vi "Text control 2 v1.7.vi"() -> ()   [LabVIEW 2016]
panel:
  in  "byte count":u32=64
  in  "Serial Settings:Serial End Mode for Reads":u16(ring)=2 items=["None", "LastBit", "TermChar"]
  in  "Timeout (ms)":u32=10000
  in  "Enable Termination\nChar (T)":bool=TRUE
  in  "Termination char\n(0xA = '\\n' = LF)\n(0xD = '\\r' = CR)":u8=13 format="%.0x"
  in  "flow control":u16(ring) items=["None"=0, "XON/XOFF"=1, "RTS/CTS"=2, "DTR/DSR"=4]
  in  "stop bits":u16(ring)=10 items=["1.0"=10, "1.5"=15, "2.0"=20]
  in  "parity":u16(ring) items=["None", "Odd", "Even", "Mark", "Space"]
  in  "data bits":u16=8 min=5 max=8 step=1
  in  "VISA resource name":refnum<visa-resource-name>="COM6"
  in  "baud rate":u32=9600
  out "Serial output":string
  out "error out":errorcluster
  in  "Units":bool
  out "Elapsed Time":dbl caption="Elapsed Time (s)"
  out "Ion vs time":cluster{"Y data in":dbl[], "X data in":dbl[]}[](graph)
  out "Ig":dbl format="%.2e"
  out "Id":dbl format="%.2e"
  out "Is":dbl format="%.2e"
  out "I vs Vg":cluster{"Y data in":dbl[], "X data in":dbl[]}[](graph)
  in  "Panel Controls 2":T1={"Emergency Stop"=refnum, "TransGraph Max"=1e-05, "Text/Graph (text=false)"=TRUE, "TransGraph Min"=1e-11} {"TransGraph Min" format="%.2e"; "TransGraph Max" format="%.2e"}
  out "Currently running:":string="#output s 0 0 0 -0.008 0.008 0.002"
  in  "Lines left to run:":string
  in  "Standby":T2
  in  "Full Reset":bool
  in  "SMU4":cluster{"on/off":bool, "Voltage":dbl} {"Voltage" min=-100.0 max=100.0 format="%.2f"}
  in  "Source/Drain Range":u8(slide)=6 max=11 scale=0.0..11.0
  in  "Source/Drain\nRange mode":u16(ring) items=["Auto", "Limited", "Fixed"]
  in  "Gate Range":u8(slide)=6 max=11 scale=0.0..11.0
  in  "Gate Range\nmode":u16(ring) items=["Auto", "Limited", "Fixed"]
  in  "Gate":T3={"Gate Start"=0.0, "Gate Stop"=2.0, "Gate Step (linear only)"=1.0, "Gate Compliance"=0.0001, "Gate PComp"=0.0, "Range mode"=0, "Range"=6} {"Range" max=11 scale=0.0..11.0; "Range mode" items=["Auto", "Limited", "Fixed"]; "Gate PComp" format="%^.2e"; "Gate Compliance" format="%^.2e"; "Gate Step (linear only)" format="%^.4e"; "Gate Stop" format="%^.4e"; "Gate Start" format="%^.4e"}
  in  "Drain 2":T4={"Drain Start"=0.0, "Drain Stop"=2.0, "Drain Compliance"=0.0001, "Drain Step"=1.0, "Drain PComp"=0.0, "Range mode"=0, "Range"=6} {"Range" max=11 scale=0.0..11.0; "Range mode" items=["Auto", "Limited", "Fixed"]; "Drain PComp" format="%^.2e"; "Drain Step" format="%^.4e"; "Drain Compliance" format="%^.2e"; "Drain Stop" format="%^.4e"; "Drain Start" format="%^.4e"}
  in  "Timings 2":T5={"integration time"=0, "Short/Long integration time"=0.00064, "hold time (sec)"=0.0, "delay time (sec)"=0.0, "Step Time (0 disables)"=0.0, "sweep method"=0, "Pulse period"=0.005, "Base voltage"=0.0, "Pulse width"=0.0005} {"Pulse width" min=0.0005 max=0.1 step=0.0001 format="%.4f"; "Base voltage" format="%^.4e"; "Pulse period" min=0.005 max=1.0 step=0.0001 format="%.4f"; "sweep method" items=["Continuous", "Pulsed"]; "Step Time (0 disables)" format="%.2f"; "delay time (sec)" format="%.4f"; "hold time (sec)" format="%.4f"; "Short/Long integration time" format="%^.0e"; "integration time" scale=0.0..2.0}
  in  "Panel Controls":T6={"Emergency Stop"=refnum, "TransGraph Max"=1e-05, "Text/Graph (text=false)"=TRUE} {"TransGraph Max" format="%.2e"}
  in  "Interrupt run":bool
  in  "Drain: Compliance":dbl=0.001 format="%.8f"
  in  "Gate: Compliance":dbl=0.001 format="%.8f"
  out "Path":path=path "C:/users/rlp38/09Apr2009LTtesting/test2.txt"
  in  "hold time /s":dbl format="%.2f"
  in  "delay time /s":dbl format="%.2f"
  in  "integration time":u32(slide) max=2 step=1 scale=0.0..2.0
  in  "Integration time (short)":dbl=0.0019 min=8e-05 max=0.0019 step=8e-05 format="%^.0e"
  in  "Integration time (long)":dbl=0.32 min=0.04 max=2.0 step=0.02 format="%.2f"
  in  "Step delay /s":dbl format="%.2f"
  in  "Program":string="#pulsedstressV d 0.03 20 0 0.5 0.0827 5\n#\n#itime s\n#gaterangemode l\n#drainrangemode l\n#pulsed on 0.05 0 0.02\n#transfer d 1 -1 -0.1 -1 -1 0\n#wait-min 1\n#transfer d 1 -1 -0.1 -1 -1 0\n#output d 0 -1 -0.5 0 -1 -0.1\n#transfer d -10 40 1 5 40 35\n#transfer d -10 40 1 5 40 35\n#output d 0 40 20 0 40 1\n#\n#\n#sample 1 0.008 221 6 0.003\n#samplei 400e-6 200 6 0.002 0.1\n#vsu2pulse -10 4\n#\n#stressV 0.016 0.03 2e-4 0.1e-3 11\n#stressI 220e-7 0.08 15\n#transfer s -1 1 0.5 -0.005 0.005 0.005\n#output s 0 0 0 -0.008 0.008 0.002\n"
  # "Syntax:\nitime [s|m|l]\ngaterangemode [a|l|f]\ndrainrangemode [a|l|f]\npulsed [on|off] PulsePeriod(sec) PulseBaseVoltage PulseONWidth(sec)\nstandby [on l off]\nwait NumMilliseconds\nwait-min NumMinutes\n# texthere = comment\ntransfer [s|d] VgStart VgStop VgStep VdStart VdStop VdStep\noutput [s|d] VgStart VgStop VgStep VdStart VdStop VdStep\nsample Vg Vd NumSamples Time(s) SampleInterval(s)\nsamplei Idg NumSamples Time(s) SampleInterval(s) VDGcompliance\n# if in doubt use SampleInterval(s) = 0.004\nstressV VG VD IGcompliance IDcompliance Duration(sec)\nstressI IDG VDGcompliance Duration(sec)\nvsu2pulse Bias Duration(s)\npulsedstressV [s|d] VEstop VgON VgOFF Period(s) PulseONwidth(s) Vd\nsample-fpp Vg Vd NumSamples Time\nresample-fpp Vg Vd\ntransfer-fpp [s|d] VgStart VgStop VgStep VdStart VdStop VdStep\noutput-fpp [s|d] VgStart VgStop VgStep VdStart VdStop VdStep\nserial SerialPortCommand"
  # "Time"
  # "Sec"
  # "Min"
  # "100 samples is approx 13s with medium integration"
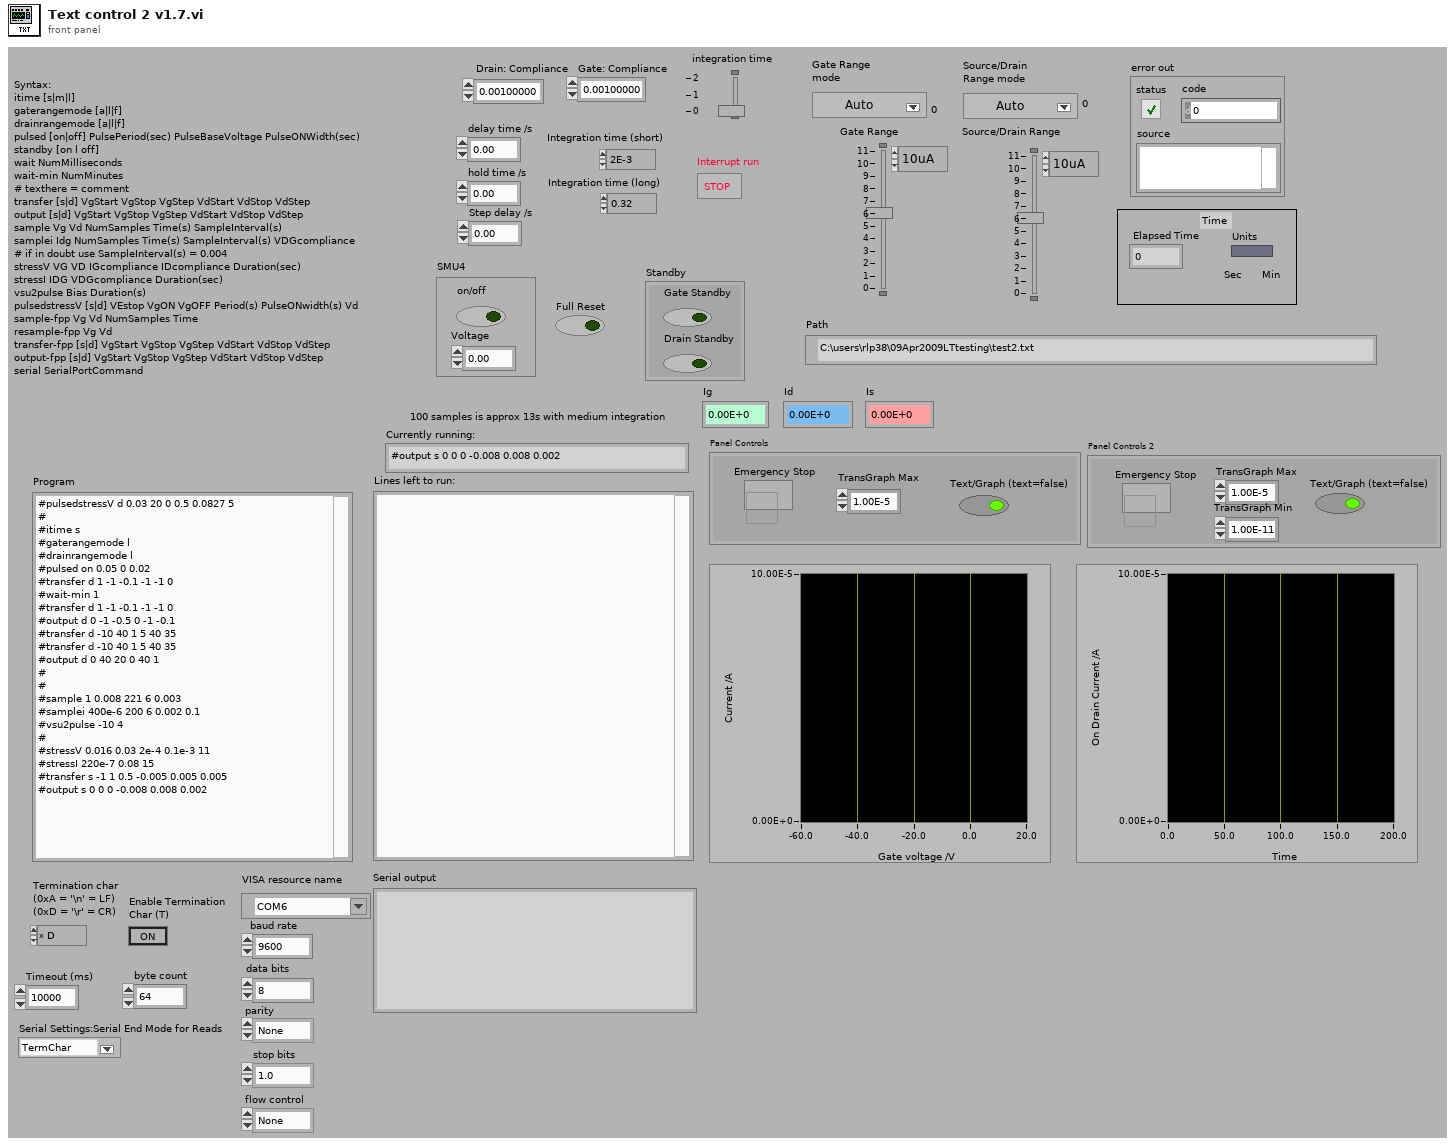
[diagram p1: front panel]
types:
  T1 = cluster{"Emergency Stop":refnum<vi>, "TransGraph Max":dbl, "Text/Graph (text=false)":bool, "TransGraph Min":dbl}
  T2 = cluster{"Gate Standby":bool, "Drain Standby":bool}
  T3 = cluster{"Gate Start":dbl, "Gate Stop":dbl, "Gate Step (linear only)":dbl, "Gate Compliance":dbl, "Gate PComp":dbl, "Range mode":u16, "Range":u8}
  T4 = cluster{"Drain Start":dbl, "Drain Stop":dbl, "Drain Compliance":dbl, "Drain Step":dbl, "Drain PComp":dbl, "Range mode":u16, "Range":u8}
  T5 = cluster{"integration time":u32, "Short/Long integration time":dbl, "hold time (sec)":dbl, "delay time (sec)":dbl, "Step Time (0 disables)":dbl, "sweep method":u16, "Pulse period":dbl, "Base voltage":dbl, "Pulse width":dbl}
  T6 = cluster{"Emergency Stop":refnum<vi>, "TransGraph Max":dbl, "Text/Graph (text=false)":bool}
  T7 = enum16{"open", "replace", "create", "open or create", "replace or create", "replace or create with confirmation"}
  T8 = cluster{"V2 Start":dbl, "V2 Step":dbl, "Number of points":i32}
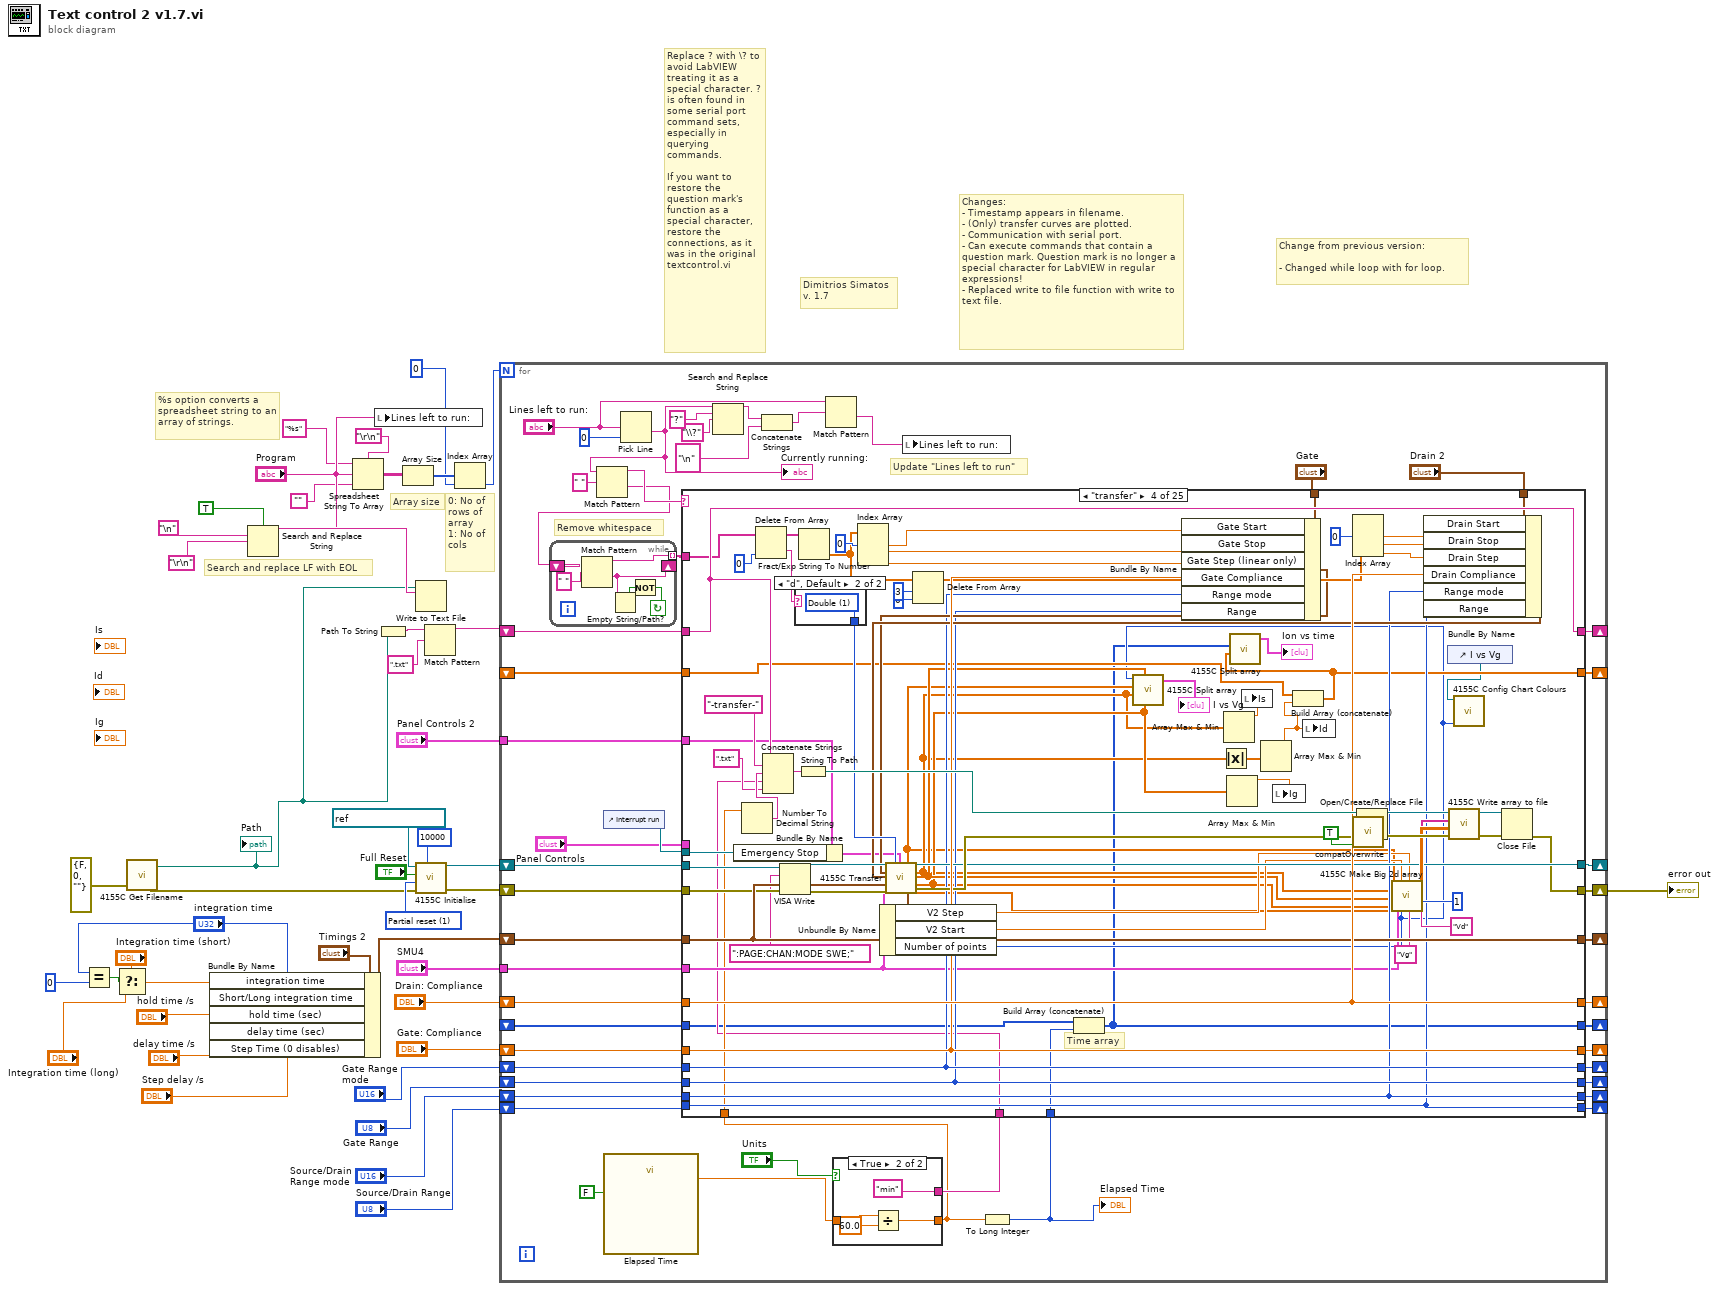
[diagram p0: block diagram]
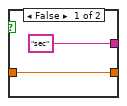
[diagram p2: hidden frame]
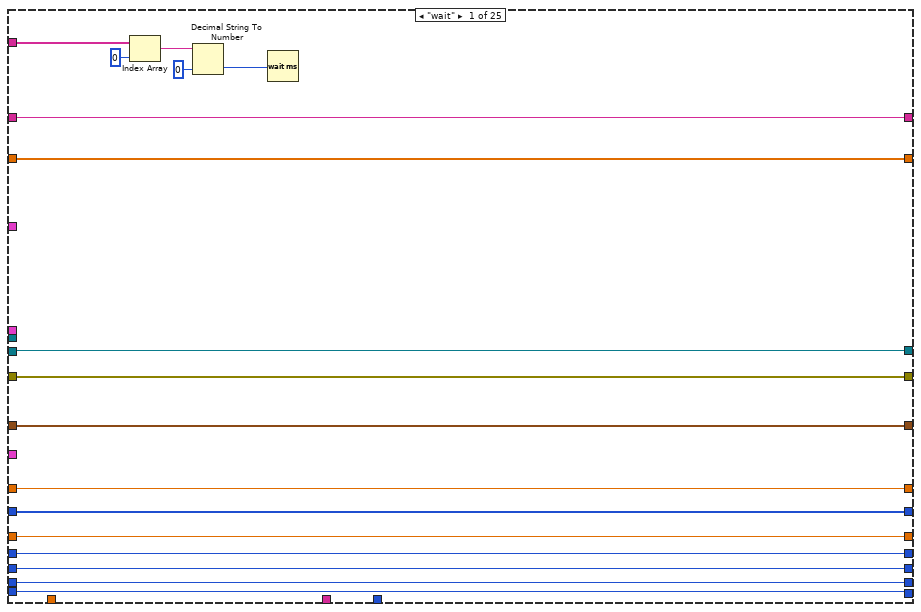
[diagram p3: hidden frame]
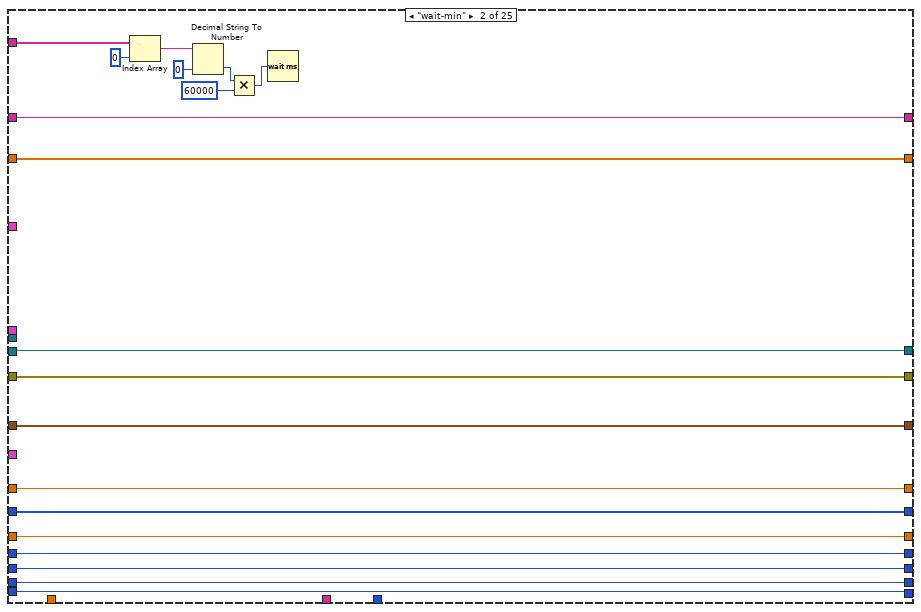
[diagram p4: hidden frame]
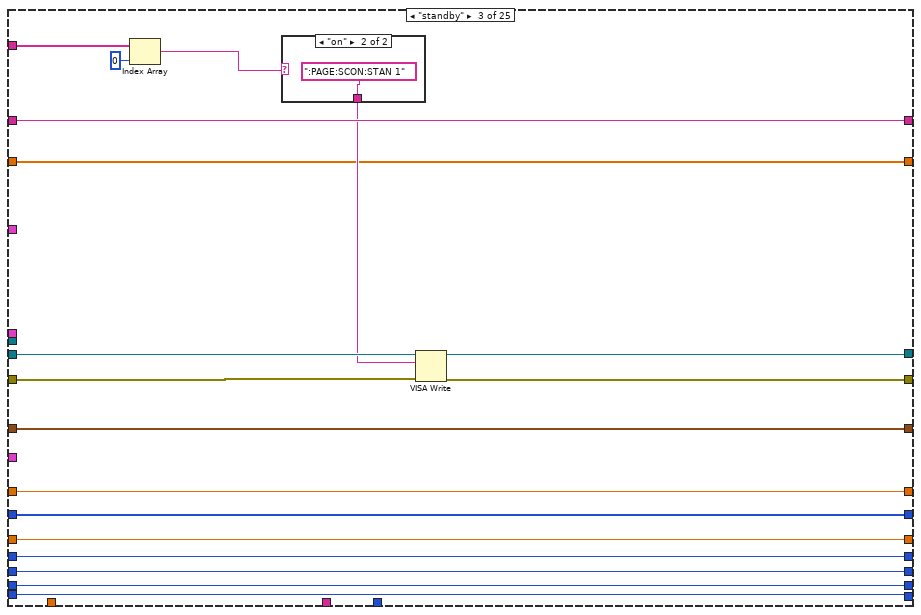
[diagram p5: hidden frame]
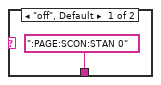
[diagram p6: hidden frame]
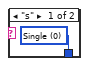
[diagram p7: hidden frame]
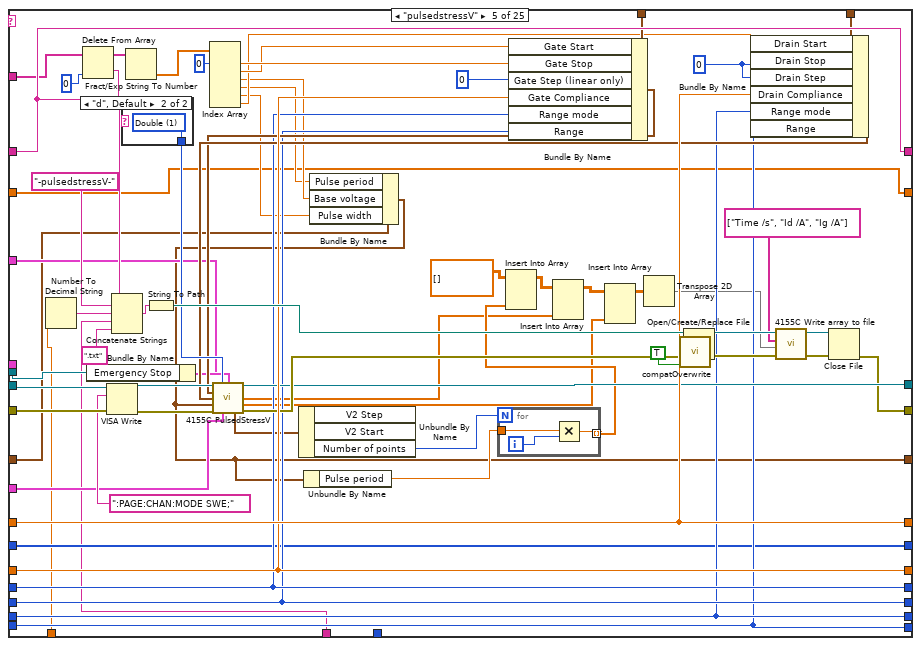
[diagram p8: hidden frame]
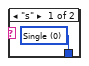
[diagram p9: hidden frame]
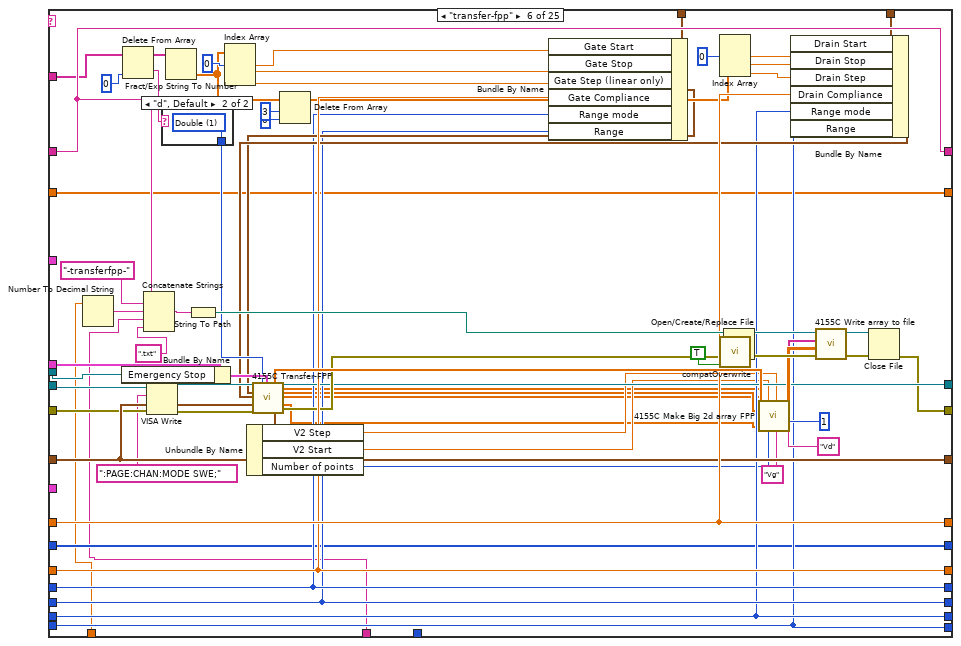
[diagram p10: hidden frame]
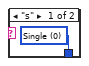
[diagram p11: hidden frame]
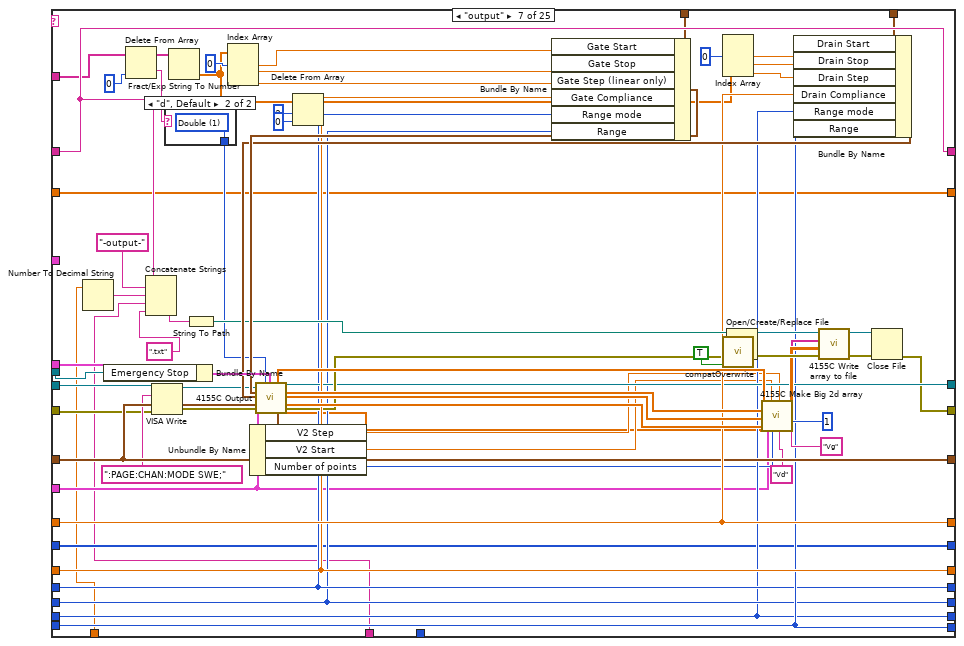
[diagram p12: hidden frame]
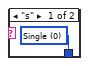
[diagram p13: hidden frame]
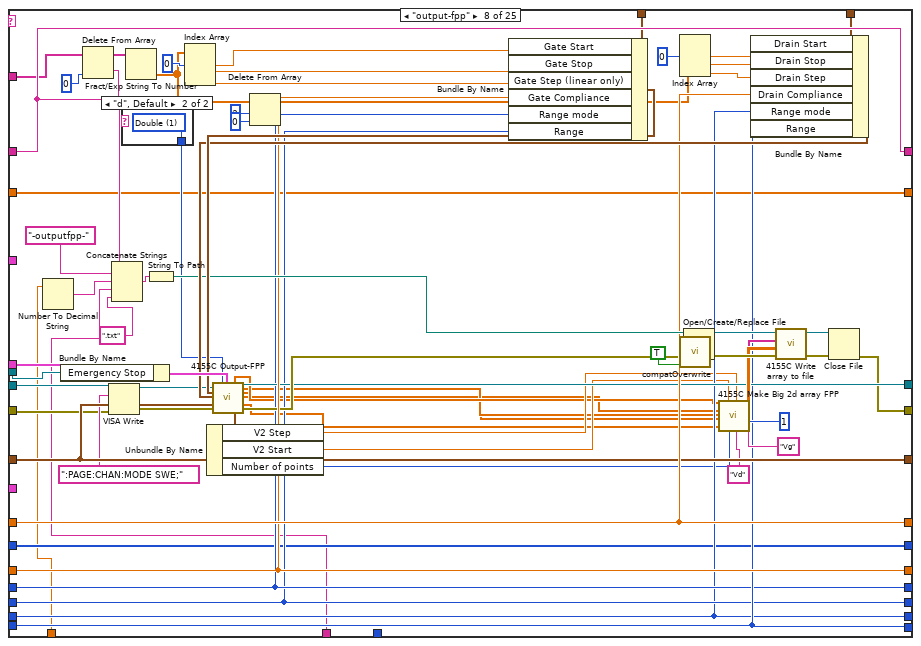
[diagram p14: hidden frame]
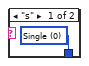
[diagram p15: hidden frame]
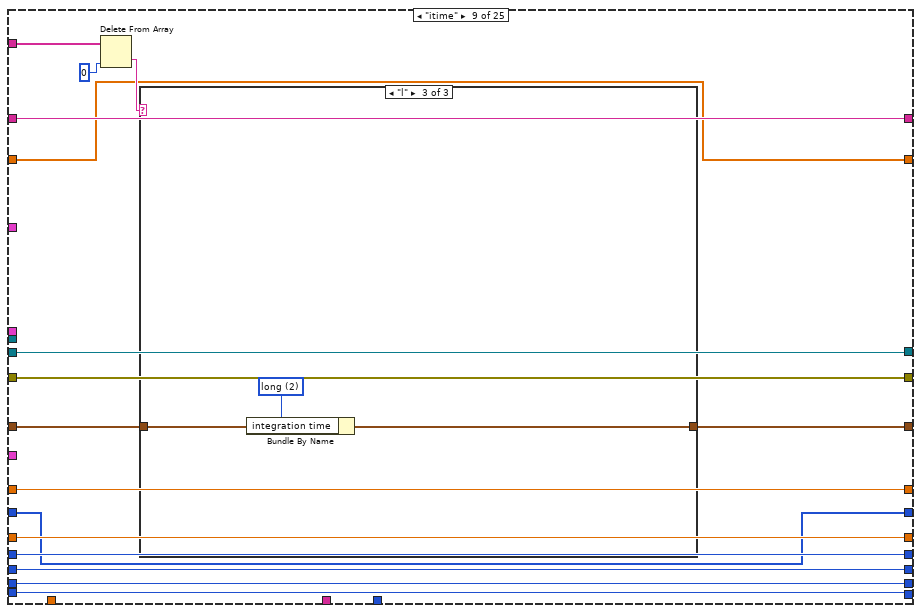
[diagram p16: hidden frame]
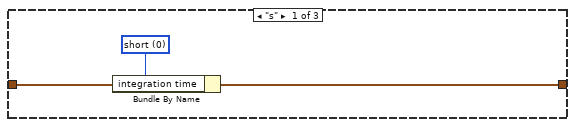
[diagram p17: hidden frame]
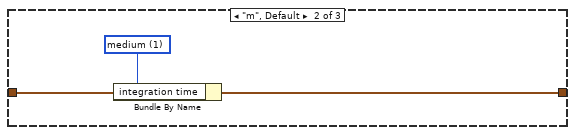
[diagram p18: hidden frame]
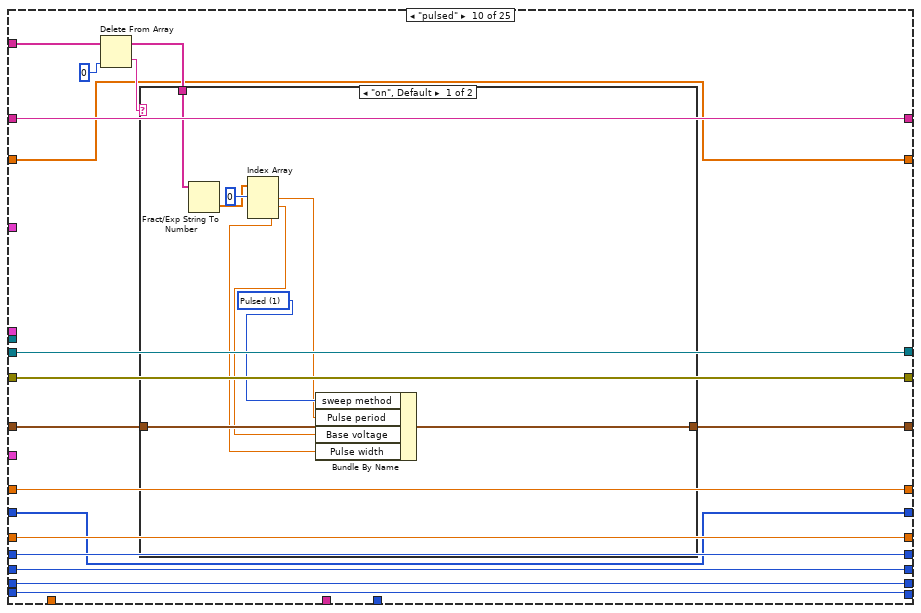
[diagram p19: hidden frame]
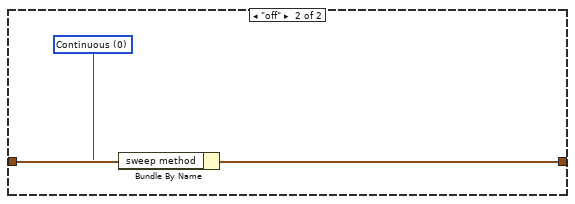
[diagram p20: hidden frame]
diagram:
  w35 = u16 1 items=["Reset All", "Partial reset"] ("Type of reset")
  # "Array size"
  # "%s option converts a spreadsheet string to an array of strings."
  # "0: No of rows of array\n1: No of cols"
  # "Change from previous version:\n\n- Changed while loop with for loop."
  # "Replace ? with \\? to avoid LabVIEW treating it as a special character. ? is often found in some serial port command sets, especially in querying commands.\n\nIf you want to restore the question mark's function as a special character, restore the connections, as it was in the original textcontrol.vi"
  # "Dimitrios Simatos\nv. 1.7"
  # "Changes:\n- Timestamp appears in filename.\n- (Only) transfer curves are plotted.\n- Communication with serial port.\n- Can execute commands that contain a question mark. Question mark is no longer a special character for LabVIEW in regular expressions!\n- Replaced write to file function with write to text file."
  # "Search and replace LF with EOL"
  n1 = Equal?(x="integration time", y=u32 0) -> (x = y?=w39:bool)
  n2 = Select(t="Integration time (short)", s=w39, f="Integration time (long)") -> (s? t:f=w43:dbl)
  n3 = call "4155C Get Filename.vi"("error in (no error)"=errorcluster {"status"=FALSE, "code"=0, "source"=""}) -> ("error out"=w30:errorcluster, "path"=w14:path)  [unwired: 2 in, 1 out]
  "Path" <- w14
  n4 = Bundle By Name(cluster="Timings 2", "integration time"="integration time", "Short/Long integration time"=w43, "hold time (sec)"="hold time /s", "delay time (sec)"="delay time /s", "Step Time (0 disables)"="Step delay /s") -> (w27:T5)
  n5 = Search and Replace String(replace all?=TRUE ("replace all? (F)"), input string="Program", search string="\n", replace string="\r\n") -> (result string=w17:string)  [unwired: 4 in, 3 out]
  n6 = Spreadsheet String To Array(delimiter (Tab)="\r\n", format string="%s", spreadsheet string="Program", array type (2D Dbl)="") -> (array=w6:string[][])
  n7 = local write "Lines left to run:"("Program") -> ()
  n8 = Path To String(path=w14) -> (string=w13:string)
  n9 = Array Size(array=w6) -> (size(s)=w5:i32[])
  n10 = Write to Text File(file (use dialog)=w14, text=w17) -> ()  [unwired: 2 in, 3 out]
  n11 = call "4155C Initialise.vi"("VISA resource name in"=refnum<visa-resource-name> "GPIB0::14::INSTR", "Reset"="Full Reset", "Type of reset"=w35, "error in (no error)"=w30, "VISA Timeout Value"=u32 10000) -> ("VISA Resource Name out"=w29:refnum<visa-resource-name>, "error out"=w28:errorcluster)
  n12 = Match Pattern(string=w13, regular expression=".txt") -> (before substring=w12:string)  [unwired: 1 in, 3 out]
  n13 = Index Array(array=w5, index=0) -> (element=w3:i32)
  n14 = for {
    N: w3 -> [_]
    tunnel: "SMU4" -> [w62]
    shift-left: "Source/Drain Range" -> [w67]
    shift-right: [w63] -> _
    shift-left: "Source/Drain\nRange mode" -> [w68]
    shift-right: [w64] -> _
    shift-left: "Gate Range" -> [w69]
    shift-right: [w65] -> _
    shift-left: "Gate Range\nmode" -> [w70]
    shift-right: [w66] -> _
    shift-left: "Gate: Compliance" -> [w81]
    shift-right: [w76] -> _
    shift-left: "Drain: Compliance" -> [w82]
    shift-right: [w77] -> _
    shift-left: w27 -> [w83]
    shift-right: [w78] -> _
    shift-left: w28 -> [w84]
    shift-right: [w79] -> w9
    shift-left: w29 -> [w85]
    shift-right: [w80] -> _
    shift-left: w12 -> [w86]
    shift-right: [w75] -> _
    tunnel: "Panel Controls 2" -> [w59]
    shift-right: [w58] -> _
    shift-left: _ -> [w57]
    shift-right: [w52] -> _
    shift-left: _ -> [w51]
    # "Remove whitespace"
    # "Update \"Lines left to run\""
    n15 = control-ref of="Interrupt run"() -> (w74:refnum<vi>)
    n16 = call "Elapsed Time"("Auto Reset"=FALSE) -> ("Elapsed Time (s)"=w53:dbl)  [unwired: 11 in, 7 out]
    n17 = Pick Line(multi-line string="Lines left to run:", line index=0) -> (output string=w48:string)  [unwired: 1 in]
    "Currently running:" <- w48
    n18 = Match Pattern(string=w48, regular expression=" ") -> (before substring=w89:string, after substring=w88:string)  [unwired: 1 in, 2 out]
    n19 = while {
      tunnel: [w100] -> w87 mode=indexing
      shift-left: w88 -> [w102]
      shift-right: [w101] -> _
      stop <- w104 continue-if-true
      n20 = Match Pattern(string=w102, regular expression=" ") -> (before substring=w100:string, after substring=w101:string)  [unwired: 1 in, 2 out]
      n21 = Empty String/Path?(string/path=w101) -> (empty?=w105:bool)
      n22 = Not(x=w105) -> (.not. x?=w104:bool)
    }
    n23 = Search and Replace String(input string=w48, search string="?", replace string="\\?") -> (result string=w46:string)  [unwired: 5 in, 3 out]
    n24 = Concatenate Strings(w46, "\n" ("Substring")) -> (w92:string)
    n25 = Match Pattern(string="Lines left to run:", regular expression=w92) -> (after substring=w60:string)  [unwired: 1 in, 3 out]
    n26 = case shown="True" "Units" {
      tunnel: ["sec" "min"] -> w54
      tunnel: [w94 w98] -> w50
      tunnel: w53 -> [w94 w97]
      frame False {
      }
      frame True {
        n27 = Divide(x=w97, y=60.0) -> (x/y=w98:dbl)
      }
    }
    n28 = local write "Lines left to run:"(w60) -> ()
    n29 = To Long Integer(number=w50) -> (32bit integer=w49:i32)
    "Elapsed Time" <- w49
    n30 = case shown="\"transfer\"" w89 {
      tunnel: w87 -> [w122 w141 w159 w223 w294 w363 w430 w505 w543 w569 w596 w621 w642 w656 _ _ w760 w821 _ w886 w930 w972 w1042 w1104 w1111]
      tunnel: w86 -> [w117 w137 w157 w231 w301 w371 w438 w513 w532 w558 w588 w614 w636 w649 w668 w710 w738 w803 w834 w873 w917 w960 w1036 w1100 w1113]
      tunnel: w85 -> [w116 w136 w148 w201 w285 w340 w406 w481 w533 w559 w589 w615 w637 w650 w673 w712 w766 w827 w838 w892 w936 w978 w1048 w1058 w1117]
      tunnel: w84 -> [w115 w135 w147 w200 w284 w339 w403 w478 w534 w560 w590 w616 w638 w651 w672 w683 w765 w826 w837 w891 w935 w977 w1047 w1057 w1116]
      tunnel: w83 -> [w114 w134 w156 w227 w260 w367 w434 w509 w542 w568 w587 w613 w635 w648 w671 w707 w729 w795 w843 w866 w910 w953 w1035 w1099 w1118]
      tunnel: w82 -> [w113 w133 w155 w229 w299 w369 w436 w511 w541 w567 w595 w620 w641 w655 w670 w692 w764 w825 w846 w890 w934 w976 w1046 w1108 w1119]
      tunnel: w81 -> [w112 w132 w154 w228 w298 w368 w435 w510 w540 w566 w594 w619 w640 w654 w669 w693 w739 w804 w845 w874 w918 w961 w1037 w1101 w1121]
      tunnel: [w116 w136 w146 w225 w296 w365 w432 w507 w533 w559 w589 w615 w637 w650 w673 w712 w730 w777 w836 w867 w911 w954 w988 w1060 w1117] -> w80
      tunnel: [w115 w135 w145 w224 w295 w364 w431 w506 w534 w560 w590 w616 w638 w651 w672 w682 w740 w778 w835 w875 w919 w962 w987 w1059 w1115] -> w79
      tunnel: [w114 w134 w156 w227 w256 w367 w434 w509 w535 w561 w587 w613 w635 w648 w671 w707 w729 w795 w843 w866 w910 w953 w1035 w1099 w1118] -> w78
      tunnel: [w113 w133 w155 w229 w299 w369 w436 w511 w541 w567 w595 w620 w641 w655 w670 w692 w764 w825 w846 w890 w934 w976 w1046 w1108 w1119] -> w77
      tunnel: [w112 w132 w154 w228 w298 w368 w435 w510 w540 w566 w594 w619 w640 w654 w669 w693 w739 w804 w845 w874 w918 w961 w1037 w1101 w1121] -> w76
      tunnel: [w117 w137 w157 w231 w301 w371 w438 w513 w532 w558 w588 w614 w636 w649 w668 w710 w738 w803 w834 w873 w917 w960 w1036 w1100 w1113] -> w75
      tunnel: w74 -> [_ _ _ w234 w305 w376 w446 w517 _ _ _ _ _ _ _ _ w735 w800 _ w872 w916 w959 w1008 w1076 _]
      tunnel: "Gate" -> [_ _ _ w210 w288 w350 w417 w492 _ _ _ _ _ _ _ _ _ _ _ _ _ _ _ _ _]
      tunnel: "Drain 2" -> [_ _ _ w209 w287 w349 w416 w491 _ _ _ _ _ _ _ _ _ _ _ _ _ _ _ _ _]
      tunnel: "Panel Controls" -> [_ _ _ _ _ w348 w415 w490 _ _ _ _ _ _ _ _ _ _ _ _ _ _ _ _ _]
      tunnel: w70 -> [w111 w131 w153 w194 w278 w333 w401 w476 w539 w565 _ w612 w634 w647 w667 w694 w725 w791 w839 w862 w906 w949 w1031 w1095 w1122]
      tunnel: w69 -> [w110 w130 w152 w193 w277 w332 w400 w475 w538 w564 w593 _ w625 w653 w666 w695 w726 w792 w840 w863 w907 w950 w1032 w1096 w1123]
      tunnel: w68 -> [w109 w129 w151 w192 w276 w331 w399 w474 w537 w563 w592 w618 w639 _ w665 w696 w727 w793 w841 w864 w908 w951 w1033 w1097 w1124]
      tunnel: w67 -> [w108 w128 w150 w191 w275 w330 w402 w477 w536 w562 w591 w617 _ w652 w664 w697 w728 w794 w842 w865 w909 w952 w1034 w1098 w1125]
      tunnel: [w111 w131 w153 w194 w278 w333 w401 w476 w539 w565 w586 w612 w634 w647 w667 w694 w725 w791 w839 w862 w906 w949 w1031 w1095 w1122] -> w66
      tunnel: [w110 w130 w152 w193 w277 w332 w400 w475 w538 w564 w593 w604 w625 w653 w666 w695 w726 w792 w840 w863 w907 w950 w1032 w1096 w1123] -> w65
      tunnel: [w109 w129 w151 w192 w276 w331 w399 w474 w537 w563 w592 w618 w639 w646 w665 w696 w727 w793 w841 w864 w908 w951 w1033 w1097 w1124] -> w64
      tunnel: [w108 w128 w150 w191 w275 w330 w402 w477 w536 w562 w591 w617 w626 w652 w664 w697 w728 w794 w842 w865 w909 w952 w1034 w1098 w1125] -> w63
      tunnel: w62 -> [_ _ _ w186 w272 _ w394 _ _ _ _ _ _ _ _ _ _ _ _ _ _ _ _ _ _]
      tunnel: w59 -> [_ _ _ w184 w271 _ _ _ _ _ _ _ _ _ _ _ _ _ _ _ _ _ _ _ _]
      tunnel: [w107 w124 w143 w173 w248 w320 w391 w463 w531 w556 w585 w603 w624 w645 w663 w678 w717 w775 w833 w851 w899 w943 w985 w1053 w1114] -> w58
      tunnel: w57 -> [w107 w124 w143 w172 w248 w320 w391 w463 w531 w556 w585 w603 w624 w645 w663 w678 w717 w775 w833 w851 w899 w943 w985 w1053 w1114]
      tunnel: w50 -> [_ _ _ w168 w245 w318 w388 w460 _ _ _ _ _ _ _ w676 w715 w772 _ w848 w896 w940 w982 w1049 _]
      tunnel: w54 -> [_ _ _ w165 w244 w316 w387 w459 _ _ _ _ _ _ _ w674 w713 w771 _ w847 w895 w939 w981 w1050 _]
      tunnel: w49 -> [_ _ _ w162 _ _ _ _ _ _ _ _ _ _ _ _ _ _ _ _ _ _ _ _ _]
      tunnel: [w106 w123 w142 w164 w247 w319 w390 w462 w530 w555 w584 w602 w623 w644 w662 w677 w716 w774 w832 w850 w898 w942 w984 w1052 w1120] -> w52
      tunnel: w51 -> [w106 w123 w142 w163 w247 w319 w390 w462 w530 w555 w584 w602 w623 w644 w662 w677 w716 w774 w832 w850 w898 w942 w984 w1052 w1120]
      frame "wait" {
        n31 = Index Array(array=w122, index=0 ("Index")) -> (element=w120:string)
        n32 = Decimal String To Number(string=w120, default (0L)=u32 0) -> (number=w119:u32)  [unwired: 1 in, 1 out]
        n33 = Wait (ms)(milliseconds to wait=w119) -> ()  [unwired: 1 out]
      }
      frame "wait-min" {
        n34 = Index Array(array=w141, index=0 ("Index")) -> (element=w139:string)
        n35 = Decimal String To Number(string=w139, default (0L)=u32 0) -> (number=w127:u32)  [unwired: 1 in, 1 out]
        n36 = Multiply(x=w127, y=u32 60000) -> (x*y=w126:u32)
        n37 = Wait (ms)(milliseconds to wait=w126) -> ()  [unwired: 1 out]
      }
      frame "standby" {
        n38 = Index Array(array=w159, index=0 ("Index")) -> (element=w149:string)
        n39 = case shown="\"on\"" w149 {
          tunnel: [":PAGE:SCON:STAN 0" ":PAGE:SCON:STAN 1"] -> w144
          frame "off", Default {
          }
          frame "on" {
          }
        }
        n40 = VISA Write(VISA resource name=w148, write buffer=w144, error in (no error)=w147) -> (VISA resource name out=w146:refnum<visa-resource-name>, error out=w145:errorcluster)  [unwired: 1 out]
      }
      frame "transfer" {
        # "Time array"
        n41 = Bundle By Name(cluster=w184, "Emergency Stop"=w234) -> (w185:T1)
        n42 = Number To Decimal String(number=w168) -> (decimal integer string=w167:string)  [unwired: 1 in]
        n43 = Delete From Array(array=w223, index=0 ("Index")) -> (deleted portion=w221:string, array with subset deleted=w220:string[])  [unwired: 1 in]
        n44 = Concatenate Strings(w231, "-transfer-" ("Prefix"), w167, w165, ".txt" ("Suffix")) -> (w233:string)
        n45 = VISA Write(VISA resource name=w201, write buffer=":PAGE:CHAN:MODE SWE;" ("write buffer (\"\")"), error in (no error)=w200) -> (VISA resource name out=w198:refnum<visa-resource-name>, error out=w199:errorcluster)  [unwired: 1 out]
        n46 = case shown="\"d\", Default" w221 {
          tunnel: [w242 w243] -> w219
          frame "s" {
            w242 = u16 0 items=["Single", "Double"] ("sweep mode")
          }
          frame "d", Default {
            w243 = u16 1 items=["Single", "Double"] ("sweep mode")
          }
        }
        n47 = String To Path(string=w233) -> (path=w230:path)
        n48 = Fract/Exp String To Number(string=w220) -> (number=w205:dbl[])  [unwired: 3 in, 1 out]
        n49 = Index Array(array=w205, index #1=0 ("Index")) -> (element #1=w218:dbl, element #2=w217:dbl, element #3=w216:dbl)  [unwired: 2 in]
        n50 = Delete From Array(array=w205, length=3 ("Length"), index=0 ("Index")) -> (array with subset deleted=w203:dbl[])  [unwired: 1 out]
        n51 = Build Array (concatenate)(w163, w162) -> (w164:i32[])
        n52 = Bundle By Name(cluster=w210, "Gate Start"=w218, "Gate Stop"=w217, "Gate Step (linear only)"=w216, "Gate Compliance"=w228, "Range mode"=w194, "Range"=w193) -> (w195:T3)
        n53 = Index Array(array=w203, index #1=0 ("Index")) -> (element #1=w213:dbl, element #2=w212:dbl, element #3=w211:dbl)  [unwired: 2 in]
        n54 = call <vilib>:"compatOverwrite.vi"("overwrite (F)"=TRUE) -> ("overwrite?"=w183:T7)
        n55 = Bundle By Name(cluster=w209, "Drain Start"=w213, "Drain Stop"=w212, "Drain Step"=w211, "Drain Compliance"=w229, "Range mode"=w192, "Range"=w191) -> (w196:T4)
        n56 = call "4155C Transfer.vi"("VISA resource name in"=w198, "Gate"=w195, "Drain"=w196, "Timings"=w227, "error in (no error)"=w199, "SMU4"=w186, "sweep mode"=w219, "Panel Controls"=w185) -> ("VG"=w174:dbl[], "Outparams"=w190:T8, "VISA Resource Name out"=w225:refnum<visa-resource-name>, "IS"=w176:dbl[], "ID"=w181:dbl[], "IG"=w177:dbl[], "error out"=w226:errorcluster, "SMU4"=w187:dbl[])  [unwired: 12 in]
        n57 = Unbundle By Name(w190) -> ("V2 Step"=w189:dbl, "V2 Start"=w188:dbl, "Number of points"=w170:i32)
        n58 = call "4155C Split array.vi"("Number of VAR2 steps"=w170, "Y2 data in"=w181, "X data in"=w174, "Y1 data in"=w176, "Y3 data in"=w177) -> ("Array of clusters"=→"I vs Vg":cluster{"Y data in":dbl[], "X data in":dbl[]}[])  [unwired: 2 in, 1 out]
        n59 = Absolute Value(x=w176) -> (abs(x)=w180:dbl[])
        n60 = Array Max & Min(array=w176) -> (max value=w178:dbl)  [unwired: 3 out]
        n61 = Array Max & Min(array=w177) -> (max value=w179:dbl)  [unwired: 3 out]
        n62 = local write "Is"(w178) -> ()
        n63 = Array Max & Min(array=w180) -> (max value=w171:dbl)  [unwired: 3 out]
        n64 = local write "Ig"(w179) -> ()
        n65 = Build Array (concatenate)(w172, w171) -> (w173:dbl[])
        n66 = call "4155C Split array.vi"("X data in"=w164, "Y1 data in"=w173) -> ("Array of clusters"=→"Ion vs time":cluster{"Y data in":dbl[], "X data in":dbl[]}[])  [unwired: 5 in, 1 out]
        n67 = local write "Id"(w171) -> ()
        n68 = Open/Create/Replace File(file path (use dialog)=w230, error in=w226, operation (0:open)=w183) -> (refnum out=w239:refnum<file>, error out=w240:errorcluster)  [unwired: 3 in, 1 out]
        n69 = call "4155C Make Big 2d array.vi"("1D Var1"=w174, "1d IS"=w176, "1d ID"=w181, "1d IG"=w177, "1d SMU4"=w187, "SMU4"=w186, "VAR2 START"=w188, "Number of VAR2 steps"=w170, "VAR2 STEP"=w189, "VAR1 Name"="Vg", "Decimal places in header"=i8 1, "VAR2 Name"="Vd") -> ("Header array"=w235:string[], "Data array"=w236:dbl[][])  [unwired: 14 in]
        n70 = control-ref of="I vs Vg"() -> (w169:refnum<vi>)
        n71 = call "4155C Write array to file.vi"("Byte Stream File Refnum"=w239, "Header"=w235, "Data Array"=w236, "error in (no error)"=w240) -> ("dup refnum"=w237:refnum<file>, "error out"=w238:errorcluster)  [unwired: 1 in]
        n72 = call "4155C Config Chart Colours.vi"("Numeric"=w170, "XY Graph 2"=w169) -> ()  [unwired: 6 in]
        n73 = Close File(refnum=w237, error in=w238) -> (error out=w224:errorcluster)  [unwired: 1 out]
      }
      frame "pulsedstressV" {
        w254 = 0
        n74 = Number To Decimal String(number=w245) -> (decimal integer string=w302:string)  [unwired: 1 in]
        n75 = Delete From Array(array=w294, index=0 ("Index")) -> (deleted portion=w292:string, array with subset deleted=w291:string[])  [unwired: 1 in]
        n76 = Bundle By Name(cluster=w271, "Emergency Stop"=w305) -> (w273:T1)
        n77 = VISA Write(VISA resource name=w285, write buffer=":PAGE:CHAN:MODE SWE;" ("write buffer (\"\")"), error in (no error)=w284) -> (VISA resource name out=w282:refnum<visa-resource-name>, error out=w283:errorcluster)  [unwired: 1 out]
        n78 = Concatenate Strings(w301, "-pulsedstressV-" ("Substring"), w302, w244, ".txt" ("Substring")) -> (w304:string)
        n79 = case shown="\"d\", Default" w292 {
          tunnel: [w314 w315] -> w290
          frame "s" {
            w314 = u16 0 items=["Single", "Double"] ("sweep mode")
          }
          frame "d", Default {
            w315 = u16 1 items=["Single", "Double"] ("sweep mode")
          }
        }
        n80 = Fract/Exp String To Number(string=w291) -> (number=w286:dbl[])  [unwired: 3 in, 1 out]
        n81 = String To Path(string=w304) -> (path=w300:path)
        n82 = Index Array(array=w286, index #1=0 ("Index")) -> (element #1=w263:dbl, element #2=w262:dbl, element #3=w259:dbl, element #4=w258:dbl, element #5=w257:dbl, element #6=w261:dbl)  [unwired: 5 in]
        n83 = Bundle By Name(cluster=w260, "Pulse period"=w258, "Base voltage"=w259, "Pulse width"=w257) -> (w256:T5)
        n84 = Unbundle By Name(w256) -> ("Pulse period"=w264:dbl)
        n85 = Bundle By Name(cluster=w288, "Gate Start"=w262, "Gate Stop"=w263, "Gate Step (linear only)"=0, "Gate Compliance"=w298, "Range mode"=w278, "Range"=w277) -> (w279:T3)
        n86 = call <vilib>:"compatOverwrite.vi"("overwrite (F)"=TRUE) -> ("overwrite?"=w249:T7)
        n87 = Bundle By Name(cluster=w287, "Drain Start"=w261, "Drain Stop"=w254, "Drain Step"=w254, "Drain Compliance"=w299, "Range mode"=w276, "Range"=w275) -> (w280:T4)
        n88 = call "4155C PulsedStressV.vi"("VISA resource name in"=w282, "sweep mode"=w290, "Panel Controls"=w273, "Gate"=w279, "Drain"=w280, "Timings"=w256, "error in (no error)"=w283, "SMU4"=w272) -> ("VISA Resource Name out"=w296:refnum<visa-resource-name>, "ID"=w252:dbl[], "IG"=w250:dbl[], "Outparams"=w274:T8, "error out"=w297:errorcluster)  [unwired: 3 in]
        n89 = Unbundle By Name(w274) -> ("Number of points"=w251:i32)  [unwired: 2 out]
        n90 = for {
          N: w251 -> [_]
          tunnel: [w311] -> w253 mode=indexing
          tunnel: w264 -> [w313]
          i -> [w312]
          n91 = Multiply(x=w313, y=w312) -> (x*y=w311:dbl)
        }
        n92 = Insert Into Array(array=dbl[][] [] ("Input Array"), new element=w253) -> (w265:dbl[][])  [unwired: 2 in]
        n93 = Insert Into Array(array=w265, new element=w252) -> (w270:dbl[][])  [unwired: 2 in]
        n94 = Insert Into Array(array=w270, new element=w250) -> (w269:dbl[][])  [unwired: 2 in]
        n95 = Transpose 2D Array(2D array=w269) -> (transposed array=w268:dbl[][])
        n96 = Open/Create/Replace File(file path (use dialog)=w300, error in=w297, operation (0:open)=w249) -> (refnum out=w308:refnum<file>, error out=w309:errorcluster)  [unwired: 3 in, 1 out]
        n97 = call "4155C Write array to file.vi"("Byte Stream File Refnum"=w308, "Header"=string[] ["Time /s", "Id /A", "Ig /A"], "Data Array"=w268, "error in (no error)"=w309) -> ("dup refnum"=w306:refnum<file>, "error out"=w307:errorcluster)  [unwired: 1 in]
        n98 = Close File(refnum=w306, error in=w307) -> (error out=w295:errorcluster)  [unwired: 1 out]
      }
      frame "transfer-fpp" {
        n99 = Number To Decimal String(number=w318) -> (decimal integer string=w372:string)  [unwired: 1 in]
        n100 = Bundle By Name(cluster=w348, "Emergency Stop"=w376) -> (w384:T6)
        n101 = Delete From Array(array=w363, index=0 ("Index")) -> (deleted portion=w361:string, array with subset deleted=w360:string[])  [unwired: 1 in]
        n102 = Concatenate Strings(w371, "-transferfpp-" ("Substring"), w372, w316, ".txt" ("Substring")) -> (w374:string)
        n103 = VISA Write(VISA resource name=w340, write buffer=":PAGE:CHAN:MODE SWE;" ("write buffer (\"\")"), error in (no error)=w339) -> (VISA resource name out=w337:refnum<visa-resource-name>, error out=w338:errorcluster)  [unwired: 1 out]
        n104 = case shown="\"d\", Default" w361 {
          tunnel: [w385 w386] -> w359
          frame "s" {
            w385 = u16 0 items=["Single", "Double"] ("sweep mode")
          }
          frame "d", Default {
            w386 = u16 1 items=["Single", "Double"] ("sweep mode")
          }
        }
        n105 = Fract/Exp String To Number(string=w360) -> (number=w344:dbl[])  [unwired: 3 in, 1 out]
        n106 = String To Path(string=w374) -> (path=w370:path)
        n107 = Index Array(array=w344, index #1=0 ("Index")) -> (element #1=w358:dbl, element #2=w357:dbl, element #3=w356:dbl)  [unwired: 2 in]
        n108 = Delete From Array(array=w344, length=3 ("Length"), index=0 ("Index")) -> (array with subset deleted=w342:dbl[])  [unwired: 1 out]
        n109 = Bundle By Name(cluster=w350, "Gate Start"=w358, "Gate Stop"=w357, "Gate Step (linear only)"=w356, "Gate Compliance"=w368, "Range mode"=w333, "Range"=w332) -> (w334:T3)
        n110 = Index Array(array=w342, index #1=0 ("Index")) -> (element #1=w353:dbl, element #2=w352:dbl, element #3=w351:dbl)  [unwired: 2 in]
        n111 = call <vilib>:"compatOverwrite.vi"("overwrite (F)"=TRUE) -> ("overwrite?"=w321:T7)
        n112 = Bundle By Name(cluster=w349, "Drain Start"=w353, "Drain Stop"=w352, "Drain Step"=w351, "Drain Compliance"=w369, "Range mode"=w331, "Range"=w330) -> (w335:T4)
        n113 = call "4155C Transfer-FPP.vi"("VISA resource name in"=w337, "Gate"=w334, "Drain"=w335, "Timings"=w367, "error in (no error)"=w338, "sweep mode"=w359, "Panel Controls"=w384) -> ("VG"=w375:dbl[], "Outparams"=w329:T8, "VISA Resource Name out"=w365:refnum<visa-resource-name>, "Vprobe2"=w325:dbl[], "ID"=w324:dbl[], "IG"=w323:dbl[], "Vprobe1"=w322:dbl[], "error out"=w366:errorcluster)  [unwired: 13 in]
        n114 = Unbundle By Name(w329) -> ("V2 Step"=w328:dbl, "V2 Start"=w327:dbl, "Number of points"=w326:i32)
        n115 = Open/Create/Replace File(file path (use dialog)=w370, error in=w366, operation (0:open)=w321) -> (refnum out=w381:refnum<file>, error out=w382:errorcluster)  [unwired: 3 in, 1 out]
        n116 = call "4155C Make Big 2d array FPP.vi"("1D Var1"=w375, "1d ID"=w324, "1d Vp2"=w325, "1d IG"=w323, "1d Vp1"=w322, "VAR2 START"=w327, "Number of VAR2 steps"=w326, "VAR2 STEP"=w328, "VAR1 Name"="Vg", "Decimal places in header"=i8 1, "VAR2 Name"="Vd") -> ("Header array"=w377:string[], "Data array"=w378:dbl[][])  [unwired: 15 in]
        n117 = call "4155C Write array to file.vi"("Byte Stream File Refnum"=w381, "Header"=w377, "Data Array"=w378, "error in (no error)"=w382) -> ("dup refnum"=w379:refnum<file>, "error out"=w380:errorcluster)  [unwired: 1 in]
        n118 = Close File(refnum=w379, error in=w380) -> (error out=w364:errorcluster)  [unwired: 1 out]
      }
      frame "output" {
        n119 = Number To Decimal String(number=w388) -> (decimal integer string=w439:string)  [unwired: 1 in]
        n120 = Bundle By Name(cluster=w415, "Emergency Stop"=w446) -> (w456:T6)
        n121 = Delete From Array(array=w430, index=0 ("Index")) -> (deleted portion=w428:string, array with subset deleted=w427:string[])  [unwired: 1 in]
        n122 = Concatenate Strings(w438, "-output-" ("Substring"), w439, w387, ".txt" ("Substring")) -> (w441:string)
        n123 = VISA Write(VISA resource name=w406, write buffer=":PAGE:CHAN:MODE SWE;" ("write buffer (\"\")"), error in (no error)=w403) -> (VISA resource name out=w405:refnum<visa-resource-name>, error out=w404:errorcluster)  [unwired: 1 out]
        n124 = case shown="\"d\", Default" w428 {
          tunnel: [w457 w458] -> w426
          frame "s" {
            w457 = u16 0 items=["Single", "Double"] ("sweep mode")
          }
          frame "d", Default {
            w458 = u16 1 items=["Single", "Double"] ("sweep mode")
          }
        }
        n125 = Fract/Exp String To Number(string=w427) -> (number=w409:dbl[])  [unwired: 3 in, 1 out]
        n126 = String To Path(string=w441) -> (path=w437:path)
        n127 = Index Array(array=w409, index #1=0 ("Index")) -> (element #1=w425:dbl, element #2=w424:dbl, element #3=w423:dbl)  [unwired: 2 in]
        n128 = Delete From Array(array=w409, length=3 ("Length"), index=0 ("Index")) -> (array with subset deleted=w408:dbl[])  [unwired: 1 out]
        n129 = Bundle By Name(cluster=w417, "Gate Start"=w425, "Gate Stop"=w424, "Gate Step (linear only)"=w423, "Gate Compliance"=w435, "Range mode"=w401, "Range"=w400) -> (w455:T3)
        n130 = Index Array(array=w408, index #1=0 ("Index")) -> (element #1=w420:dbl, element #2=w419:dbl, element #3=w418:dbl)  [unwired: 2 in]
        n131 = call <vilib>:"compatOverwrite.vi"("overwrite (F)"=TRUE) -> ("overwrite?"=w392:T7)
        n132 = Bundle By Name(cluster=w416, "Drain Start"=w420, "Drain Stop"=w419, "Drain Step"=w418, "Drain Compliance"=w436, "Range mode"=w399, "Range"=w402) -> (w454:T4)
        n133 = call "4155C Output.vi"("VISA resource name in"=w405, "Gate"=w455, "Drain"=w454, "Timings"=w434, "error in (no error)"=w404, "SMU4"=w394, "sweep mode"=w426, "Panel controls"=w456) -> ("VD"=w442:dbl[], "Outparams"=w397:T8, "VISA Resource Name out"=w432:refnum<visa-resource-name>, "IS"=w445:dbl[], "ID"=w444:dbl[], "IG"=w443:dbl[], "error out"=w433:errorcluster, "SMU4"=w393:dbl[])  [unwired: 12 in]
        n134 = Unbundle By Name(w397) -> ("V2 Step"=w398:dbl, "V2 Start"=w396:dbl, "Number of points"=w395:i32)
        n135 = Open/Create/Replace File(file path (use dialog)=w437, error in=w433, operation (0:open)=w392) -> (refnum out=w451:refnum<file>, error out=w452:errorcluster)  [unwired: 3 in, 1 out]
        n136 = call "4155C Make Big 2d array.vi"("1D Var1"=w442, "1d IS"=w445, "1d ID"=w444, "1d IG"=w443, "1d SMU4"=w393, "SMU4"=w394, "VAR2 START"=w396, "Number of VAR2 steps"=w395, "VAR2 STEP"=w398, "VAR1 Name"="Vd", "Decimal places in header"=i8 1, "VAR2 Name"="Vg") -> ("Header array"=w447:string[], "Data array"=w448:dbl[][])  [unwired: 14 in]
        n137 = call "4155C Write array to file.vi"("Byte Stream File Refnum"=w451, "Header"=w447, "Data Array"=w448, "error in (no error)"=w452) -> ("dup refnum"=w449:refnum<file>, "error out"=w450:errorcluster)  [unwired: 1 in]
        n138 = Close File(refnum=w449, error in=w450) -> (error out=w431:errorcluster)  [unwired: 1 out]
      }
      frame "output-fpp" {
        n139 = Number To Decimal String(number=w460) -> (decimal integer string=w514:string)  [unwired: 1 in]
        n140 = Bundle By Name(cluster=w490, "Emergency Stop"=w517) -> (w527:T6)
        n141 = Delete From Array(array=w505, index=0 ("Index")) -> (deleted portion=w503:string, array with subset deleted=w502:string[])  [unwired: 1 in]
        n142 = VISA Write(VISA resource name=w481, write buffer=":PAGE:CHAN:MODE SWE;" ("write buffer (\"\")"), error in (no error)=w478) -> (VISA resource name out=w480:refnum<visa-resource-name>, error out=w479:errorcluster)  [unwired: 1 out]
        n143 = Concatenate Strings(w513, "-outputfpp-" ("Substring"), w514, w459, ".txt" ("Substring")) -> (w516:string)
        n144 = case shown="\"d\", Default" w503 {
          tunnel: [w528 w529] -> w501
          frame "s" {
            w528 = u16 0 items=["Single", "Double"] ("sweep mode")
          }
          frame "d", Default {
            w529 = u16 1 items=["Single", "Double"] ("sweep mode")
          }
        }
        n145 = Fract/Exp String To Number(string=w502) -> (number=w484:dbl[])  [unwired: 3 in, 1 out]
        n146 = String To Path(string=w516) -> (path=w512:path)
        n147 = Index Array(array=w484, index #1=0 ("Index")) -> (element #1=w500:dbl, element #2=w499:dbl, element #3=w498:dbl)  [unwired: 2 in]
        n148 = Delete From Array(array=w484, length=3 ("Length"), index=0 ("Index")) -> (array with subset deleted=w483:dbl[])  [unwired: 1 out]
        n149 = Bundle By Name(cluster=w492, "Gate Start"=w500, "Gate Stop"=w499, "Gate Step (linear only)"=w498, "Gate Compliance"=w510, "Range mode"=w476, "Range"=w475) -> (w526:T3)
        n150 = Index Array(array=w483, index #1=0 ("Index")) -> (element #1=w495:dbl, element #2=w494:dbl, element #3=w493:dbl)  [unwired: 2 in]
        n151 = call <vilib>:"compatOverwrite.vi"("overwrite (F)"=TRUE) -> ("overwrite?"=w464:T7)
        n152 = Bundle By Name(cluster=w491, "Drain Start"=w495, "Drain Stop"=w494, "Drain Step"=w493, "Drain Compliance"=w511, "Range mode"=w474, "Range"=w477) -> (w525:T4)
        n153 = call "4155C Output-FPP.vi"("VISA resource name in"=w480, "Gate"=w526, "Drain"=w525, "Timings"=w509, "error in (no error)"=w479, "sweep mode"=w501, "Panel controls"=w527) -> ("VD"=w469:dbl[], "Outparams"=w472:T8, "VISA Resource Name out"=w507:refnum<visa-resource-name>, "Vprobe2"=w468:dbl[], "ID"=w467:dbl[], "IG"=w466:dbl[], "Vprobe1"=w465:dbl[], "error out"=w508:errorcluster)  [unwired: 13 in]
        n154 = Unbundle By Name(w472) -> ("V2 Step"=w473:dbl, "V2 Start"=w471:dbl, "Number of points"=w470:i32)
        n155 = Open/Create/Replace File(file path (use dialog)=w512, error in=w508, operation (0:open)=w464) -> (refnum out=w522:refnum<file>, error out=w523:errorcluster)  [unwired: 3 in, 1 out]
        n156 = call "4155C Make Big 2d array FPP.vi"("1D Var1"=w469, "1d ID"=w467, "1d Vp2"=w468, "1d IG"=w466, "1d Vp1"=w465, "VAR2 START"=w471, "Number of VAR2 steps"=w470, "VAR2 STEP"=w473, "VAR1 Name"="Vd", "Decimal places in header"=i8 1, "VAR2 Name"="Vg") -> ("Header array"=w518:string[], "Data array"=w519:dbl[][])  [unwired: 15 in]
        n157 = call "4155C Write array to file.vi"("Byte Stream File Refnum"=w522, "Header"=w518, "Data Array"=w519, "error in (no error)"=w523) -> ("dup refnum"=w520:refnum<file>, "error out"=w521:errorcluster)  [unwired: 1 in]
        n158 = Close File(refnum=w520, error in=w521) -> (error out=w506:errorcluster)  [unwired: 1 out]
      }
      frame "itime" {
        n159 = Delete From Array(array=w543, index=0 ("Index")) -> (deleted portion=w544:string)  [unwired: 1 in, 1 out]
        n160 = case shown="\"l\"" w544 {
          tunnel: w542 -> [w548 w550 w553]
          tunnel: [w547 w549 w552] -> w535
          frame "s" {
            w546 = u32 0 items=["short  ", "medium  ", "long  "] ("integration time 2")
            n161 = Bundle By Name(cluster=w548, "integration time"=w546) -> (w547:T5)
          }
          frame "m", Default {
            w551 = u32 1 items=["short  ", "medium  ", "long  "] ("integration time 2")
            n162 = Bundle By Name(cluster=w550, "integration time"=w551) -> (w549:T5)
          }
          frame "l" {
            w554 = u32 2 items=["short  ", "medium  ", "long  "] ("integration time 2")
            n163 = Bundle By Name(cluster=w553, "integration time"=w554) -> (w552:T5)
          }
        }
      }
      frame "pulsed" {
        n164 = Delete From Array(array=w569, index=0 ("Index")) -> (deleted portion=w570:string, array with subset deleted=w557:string[])  [unwired: 1 in]
        n165 = case shown="\"on\", Default" w570 {
          tunnel: w568 -> [w580 w583]
          tunnel: [w579 w582] -> w561
          tunnel: w557 -> [w577 _]
          frame "on", Default {
            w578 = u16 1 items=["Continuous", "Pulsed"] ("sweep method")
            n166 = Fract/Exp String To Number(string=w577) -> (number=w575:dbl[])  [unwired: 3 in, 1 out]
            n167 = Index Array(array=w575, index #1=0 ("Index")) -> (element #1=w574:dbl, element #2=w573:dbl, element #3=w572:dbl)  [unwired: 2 in]
            n168 = Bundle By Name(cluster=w580, "sweep method"=w578, "Pulse period"=w574, "Base voltage"=w573, "Pulse width"=w572) -> (w579:T5)
          }
          frame "off" {
            w581 = u16 0 items=["Continuous", "Pulsed"] ("sweep method")
            n169 = Bundle By Name(cluster=w583, "sweep method"=w581) -> (w582:T5)
          }
        }
      }
      frame "gaterangemode" {
        n170 = Delete From Array(array=w596, index=0 ("Index")) -> (deleted portion=w597:string)  [unwired: 1 in, 1 out]
        n171 = case shown="\"f\"" w597 {
          tunnel: [w599 w600 w601] -> w586
          frame "a", Default {
            w599 = u16 0 items=["Auto", "Limited", "Fixed"] ("Gate Range\nmode 2")
          }
          frame "f" {
            w600 = u16 2 items=["Auto", "Limited", "Fixed"] ("Gate Range\nmode 2")
          }
          frame "l" {
            w601 = u16 1 items=["Auto", "Limited", "Fixed"] ("Gate Range\nmode 2")
          }
        }
      }
      frame "gaterange" {
        (unwired) u8 11 items=["10fA  ", "100fA  ", "1nA  ", "10nA", "100nA", "1uA", "10uA", "100uA", "1mA", "10mA", "100mA", "1A"] ("Gate Range 2")
        n172 = Delete From Array(array=w621, index=0 ("Index")) -> (deleted portion=w611:string)  [unwired: 1 in, 1 out]
        n173 = Scan Value(string=w611, format string="") -> (value=w609:dbl)  [unwired: 1 in, 1 out]
        n174 = Logarithm Base 10(1:w609) -> (0:w608:dbl)
        n175 = Round To Nearest(number=w608) -> (nearest integer value=w607:dbl)
        n176 = Add(x=w607, y=11.0) -> (x+y=w605:dbl)
        n177 = To Unsigned Byte Integer(number=w605) -> (unsigned 8bit integer=w604:u8)
      }
      frame "drainrange" {
        (unwired) u8 11 items=["10fA  ", "100fA  ", "1nA  ", "10nA", "100nA", "1uA", "10uA", "100uA", "1mA", "10mA", "100mA", "1A"] ("Gate Range 2")
        n178 = Delete From Array(array=w642, index=0 ("Index")) -> (deleted portion=w633:string)  [unwired: 1 in, 1 out]
        n179 = Scan Value(string=w633, format string="") -> (value=w631:dbl)  [unwired: 1 in, 1 out]
        n180 = Logarithm Base 10(1:w631) -> (0:w630:dbl)
        n181 = Round To Nearest(number=w630) -> (nearest integer value=w629:dbl)
        n182 = Add(x=w629, y=11.0) -> (x+y=w627:dbl)
        n183 = To Unsigned Byte Integer(number=w627) -> (unsigned 8bit integer=w626:u8)
      }
      frame "drainrangemode" {
        n184 = Delete From Array(array=w656, index=0 ("Index")) -> (deleted portion=w657:string)  [unwired: 1 in, 1 out]
        n185 = case shown="\"f\"" w657 {
          tunnel: [w659 w660 w661] -> w646
          frame "a", Default {
            w659 = u16 0 items=["Auto", "Limited", "Fixed"] ("Gate Range\nmode 2")
          }
          frame "f" {
            w660 = u16 2 items=["Auto", "Limited", "Fixed"] ("Gate Range\nmode 2")
          }
          frame "l" {
            w661 = u16 1 items=["Auto", "Limited", "Fixed"] ("Gate Range\nmode 2")
          }
        }
      }
      frame "Error", Default {
      }
      frame "logfile" {
        n186 = Number To Decimal String(number=w676) -> (decimal integer string=w711:string)  [unwired: 1 in]
        n187 = Concatenate Strings(w710, "logfile" ("Substring"), w711, w674, ".txt" ("Substring")) -> (w708:string)
        n188 = String To Path(string=w708) -> (path=w681:path)
        n189 = Unbundle(w707) -> ("integration time"=w706:u32, "Short/Long integration time"=w705:dbl, "hold time (sec)"=w704:dbl, "delay time (sec)"=w703:dbl, "Step Time (0 disables)"=w702:dbl, "sweep method"=w701:u16, "Pulse period"=w700:dbl, "Base voltage"=w699:dbl, "Pulse width"=w698:dbl)
        n190 = Build Array(w706, w705, w704, w703, w702, w701, w700, w699, w698, w692, w693, w694, w695, w696, w697) -> (w685:dbl[])
        n191 = Insert Into Array(array=dbl[][] [] ("Input Array"), new element=w685) -> (w684:dbl[][])  [unwired: 2 in]
        n192 = call <vilib>:"compatOverwrite.vi"("overwrite (F)"=TRUE) -> ("overwrite?"=w679:T7)
        n193 = Open/Create/Replace File(file path (use dialog)=w681, error in=w683, operation (0:open)=w679) -> (refnum out=w689:refnum<file>, error out=w688:errorcluster)  [unwired: 3 in, 1 out]
        n194 = call "4155C Write array to file.vi"("Byte Stream File Refnum"=w689, "Header"=string[] ["Int Time", "Short/Long Itime", "Hold time", "Delay time", "Step time", "Sweep method", "Pulse period", "Base Voltage", "Pulse width", "Drain compliance", "Gate compliance", "Gate range mode", "Gate range", "S/D range mode", "S/D range"], "Data Array"=w684, "error in (no error)"=w688) -> ("dup refnum"=w691:refnum<file>, "error out"=w690:errorcluster)  [unwired: 1 in]
        n195 = Close File(refnum=w691, error in=w690) -> (error out=w682:errorcluster)  [unwired: 1 out]
      }
      frame "sample" {
        n196 = Number To Decimal String(number=w715) -> (decimal integer string=w763:string)  [unwired: 1 in]
        n197 = Fract/Exp String To Number(string=w760) -> (number=w721:dbl[])  [unwired: 3 in, 1 out]
        n198 = Concatenate Strings(w738, "-sample-" ("Substring"), w763, w713, ".txt" ("Substring")) -> (w761:string)
        n199 = String To Path(string=w761) -> (path=w742:path)
        n200 = Index Array(array=w721, index=0 ("Index")) -> (element=w758:dbl)
        n201 = Index Array(array=w721, index=2 ("Index")) -> (element=w754:dbl)
        n202 = Index Array(array=w721, index=3 ("Index")) -> (element=w723:dbl)
        n203 = Index Array(array=w721, index=4 ("Index")) -> (element=w720:dbl)
        n204 = call "4155C Config Sampling Measurements.vi"("Sampling interval"=w720, "Sample time"=w723, "Display on/off"=TRUE, "Timings"=w729, "Num Points"=w754, "error in (no error)"=w765, "Drain Compliance"=w764, "Gate Compliance"=w739, "VISA session"=w766) -> ("error out"=w767:errorcluster, "dup VISA resource name"=w768:refnum<visa-resource-name>)  [unwired: 1 in]
        n205 = Index Array(array=w721, index=1 ("Index")) -> (element=w755:dbl)
        n206 = call "4155C Take Sample.vi"("Emergency Stop"=w735, "error in (no error)"=w767, "Vd"=w755, "Vg"=w758, "VISA resource name in"=w768) -> ("error out"=w733:errorcluster, "Id"=w770:dbl[], "Ig"=w744:dbl[], "VISA Resource Name out"=w731:refnum<visa-resource-name>, "Is"=w769:dbl[], "Time"=w748:dbl[])  [unwired: 1 in]
        n207 = Insert Into Array(array=dbl[][] [] ("Input Array"), new element=w748) -> (w747:dbl[][])  [unwired: 2 in]
        n208 = Insert Into Array(array=w747, new element=w744) -> (w746:dbl[][])  [unwired: 2 in]
        n209 = Insert Into Array(array=w746, new element=w770) -> (w745:dbl[][])  [unwired: 2 in]
        n210 = VISA Write(VISA resource name=w731, write buffer=":DISP ON" ("write buffer (\"\")"), error in (no error)=w733) -> (VISA resource name out=w730:refnum<visa-resource-name>, error out=w732:errorcluster)  [unwired: 1 out]
        n211 = Insert Into Array(array=w745, new element=w769) -> (w737:dbl[][])  [unwired: 2 in]
        n212 = Transpose 2D Array(2D array=w737) -> (transposed array=w736:dbl[][])
        n213 = call <vilib>:"compatOverwrite.vi"("overwrite (F)"=TRUE) -> ("overwrite?"=w718:T7)
        n214 = Open/Create/Replace File(file path (use dialog)=w742, error in=w732, operation (0:open)=w718) -> (refnum out=w751:refnum<file>, error out=w750:errorcluster)  [unwired: 3 in, 1 out]
        n215 = call "4155C Write array to file.vi"("Byte Stream File Refnum"=w751, "Header"=string[] ["Time /s", "Ig /A", "Id /A", "Is /A"], "Data Array"=w736, "error in (no error)"=w750) -> ("dup refnum"=w753:refnum<file>, "error out"=w752:errorcluster)  [unwired: 1 in]
        n216 = Close File(refnum=w753, error in=w752) -> (error out=w740:errorcluster)  [unwired: 1 out]
      }
      frame "samplei" {
        n217 = Number To Decimal String(number=w772) -> (decimal integer string=w824:string)  [unwired: 1 in]
        n218 = Fract/Exp String To Number(string=w821) -> (number=w788:dbl[])  [unwired: 3 in, 1 out]
        n219 = Concatenate Strings(w803, "-samplei-" ("Substring"), w824, w771, ".txt" ("Substring")) -> (w822:string)
        n220 = String To Path(string=w822) -> (path=w806:path)
        n221 = Index Array(array=w788, index=4 ("Index")) -> (element=w782:dbl)
        n222 = Index Array(array=w788, index=3 ("Index")) -> (element=w783:dbl)
        n223 = Index Array(array=w788, index=1 ("Index")) -> (element=w785:dbl)
        n224 = Index Array(array=w788, index=0 ("Index")) -> (element=w786:dbl)
        n225 = Index Array(array=w788, index=2 ("Index")) -> (element=w784:dbl)
        n226 = call "4155C Config SamplingI Measurements.vi"("Sample time"=w784, "Display on/off"=TRUE, "Timings"=w795, "Num Points"=w785, "error in (no error)"=w826, "Sampling interval"=w783, "VISA session"=w827) -> ("error out"=w828:errorcluster, "dup VISA resource name"=w829:refnum<visa-resource-name>)  [unwired: 3 in]
        n227 = call "4155C Take SampleI.vi"("Emergency Stop"=w800, "error in (no error)"=w828, "Idg 2"=w786, "Vdg compliance 2"=w782, "VISA resource name in"=w829) -> ("error out"=w798:errorcluster, "Idg"=w831:dbl[], "Vdg"=w808:dbl[], "VISA Resource Name out"=w796:refnum<visa-resource-name>, "Is"=w830:dbl[], "Time"=w812:dbl[])  [unwired: 1 in]
        n228 = Insert Into Array(array=dbl[][] [] ("Input Array"), new element=w812) -> (w811:dbl[][])  [unwired: 2 in]
        n229 = Insert Into Array(array=w811, new element=w808) -> (w810:dbl[][])  [unwired: 2 in]
        n230 = Insert Into Array(array=w810, new element=w831) -> (w809:dbl[][])  [unwired: 2 in]
        n231 = VISA Write(VISA resource name=w796, write buffer=":DISP ON" ("write buffer (\"\")"), error in (no error)=w798) -> (VISA resource name out=w781:refnum<visa-resource-name>, error out=w797:errorcluster)  [unwired: 1 out]
        n232 = Insert Into Array(array=w809, new element=w830) -> (w802:dbl[][])  [unwired: 2 in]
        n233 = Transpose 2D Array(2D array=w802) -> (transposed array=w801:dbl[][])
        n234 = call <vilib>:"compatOverwrite.vi"("overwrite (F)"=TRUE) -> ("overwrite?"=w776:T7)
        n235 = Open/Create/Replace File(file path (use dialog)=w806, error in=w797, operation (0:open)=w776) -> (refnum out=w815:refnum<file>, error out=w814:errorcluster)  [unwired: 3 in, 1 out]
        n236 = call "4155C Write array to file.vi"("Byte Stream File Refnum"=w815, "Header"=string[] ["Time /s", "Vdg /V", "Idg /A", "Is /A"], "Data Array"=w801, "error in (no error)"=w814) -> ("dup refnum"=w817:refnum<file>, "error out"=w816:errorcluster)  [unwired: 1 in]
        n237 = Close File(refnum=w817, error in=w816) -> (error out=w779:errorcluster)  [unwired: 1 out]
        n238 = VISA Write(VISA resource name=w781, write buffer=";:PAGE:SCON:STAN OFF;:PAGE:CHAN:VSU2:DIS;" ("write buffer (\"\")"), error in (no error)=w779) -> (VISA resource name out=w777:refnum<visa-resource-name>, error out=w778:errorcluster)  [unwired: 1 out]
      }
      frame "#" {
        n239 = VISA Write(VISA resource name=w838, write buffer=":DISP ON" ("write buffer (\"\")"), error in (no error)=w837) -> (VISA resource name out=w836:refnum<visa-resource-name>, error out=w835:errorcluster)  [unwired: 1 out]
      }
      frame "stressV" {
        n240 = Number To Decimal String(number=w848) -> (decimal integer string=w889:string)  [unwired: 1 in]
        n241 = Fract/Exp String To Number(string=w886) -> (number=w859:dbl[])  [unwired: 3 in, 1 out]
        n242 = Concatenate Strings(w873, "-stressV-" ("Substring"), w889, w847, ".txt" ("Substring")) -> (w887:string)
        n243 = String To Path(string=w887) -> (path=w877:path)
        n244 = Index Array(array=w859, index=3 ("Index")) -> (element=w856:dbl)
        n245 = Index Array(array=w859, index=1 ("Index")) -> (element=w854:dbl)
        n246 = Index Array(array=w859, index=0 ("Index")) -> (element=w853:dbl)
        n247 = Index Array(array=w859, index=4 ("Index")) -> (element=w858:dbl)
        n248 = Index Array(array=w859, index=2 ("Index")) -> (element=w855:dbl)
        n249 = call "4155C Config V Stress.vi"("VISA session"=w892, "ID compliance"=w856, "VD"=w854, "VG"=w853, "IG compliance"=w855, "error in (no error)"=w891, "Display on/off"=TRUE) -> ("dup VISA resource name"=w894:refnum<visa-resource-name>, "error out"=w893:errorcluster)
        n250 = call "4155C Apply Stress.vi"("error in (no error)"=w893, "Duration"=w858, "Emergency Stop"=w872, "VISA resource name in"=w894) -> ("error out"=w870:errorcluster, "VISA Resource Name out"=w868:refnum<visa-resource-name>)
        n251 = VISA Write(VISA resource name=w868, write buffer=":DISP ON" ("write buffer (\"\")"), error in (no error)=w870) -> (VISA resource name out=w867:refnum<visa-resource-name>, error out=w869:errorcluster)  [unwired: 1 out]
        n252 = call <vilib>:"compatOverwrite.vi"("overwrite (F)"=TRUE) -> ("overwrite?"=w852:T7)
        n253 = Open/Create/Replace File(file path (use dialog)=w877, error in=w869, operation (0:open)=w852) -> (refnum out=w880:refnum<file>, error out=w879:errorcluster)  [unwired: 3 in, 1 out]
        n254 = call "4155C Write array to file.vi"("Byte Stream File Refnum"=w880, "Header"=string[] ["V stress completed successfully", ""], "error in (no error)"=w879) -> ("dup refnum"=w882:refnum<file>, "error out"=w881:errorcluster)  [unwired: 2 in]
        n255 = Close File(refnum=w882, error in=w881) -> (error out=w875:errorcluster)  [unwired: 1 out]
      }
      frame "stressI" {
        n256 = Number To Decimal String(number=w896) -> (decimal integer string=w933:string)  [unwired: 1 in]
        n257 = Fract/Exp String To Number(string=w930) -> (number=w905:dbl[])  [unwired: 3 in, 1 out]
        n258 = Concatenate Strings(w917, "-stressI-" ("Substring"), w933, w895, ".txt" ("Substring")) -> (w931:string)
        n259 = String To Path(string=w931) -> (path=w921:path)
        n260 = Index Array(array=w905, index=1 ("Index")) -> (element=w901:dbl)
        n261 = Index Array(array=w905, index=0 ("Index")) -> (element=w902:dbl)
        n262 = call "4155C Config I Stress.vi"("VISA session"=w936, "IDG"=w902, "VDG compliance"=w901, "error in (no error)"=w935, "Display on/off"=TRUE) -> ("dup VISA resource name"=w938:refnum<visa-resource-name>, "error out"=w937:errorcluster)
        n263 = Index Array(array=w905, index=2 ("Index")) -> (element=w903:dbl)
        n264 = call "4155C Apply Stress.vi"("error in (no error)"=w937, "Duration"=w903, "Emergency Stop"=w916, "VISA resource name in"=w938) -> ("error out"=w914:errorcluster, "VISA Resource Name out"=w912:refnum<visa-resource-name>)
        n265 = VISA Write(VISA resource name=w912, write buffer=":DISP ON" ("write buffer (\"\")"), error in (no error)=w914) -> (VISA resource name out=w911:refnum<visa-resource-name>, error out=w913:errorcluster)  [unwired: 1 out]
        n266 = call <vilib>:"compatOverwrite.vi"("overwrite (F)"=TRUE) -> ("overwrite?"=w900:T7)
        n267 = Open/Create/Replace File(file path (use dialog)=w921, error in=w913, operation (0:open)=w900) -> (refnum out=w924:refnum<file>, error out=w923:errorcluster)  [unwired: 3 in, 1 out]
        n268 = call "4155C Write array to file.vi"("Byte Stream File Refnum"=w924, "Header"=string[] ["I stress completed successfully", ""], "error in (no error)"=w923) -> ("dup refnum"=w926:refnum<file>, "error out"=w925:errorcluster)  [unwired: 2 in]
        n269 = Close File(refnum=w926, error in=w925) -> (error out=w919:errorcluster)  [unwired: 1 out]
      }
      frame "vsu2pulse" {
        n270 = Number To Decimal String(number=w940) -> (decimal integer string=w975:string)  [unwired: 1 in]
        n271 = Fract/Exp String To Number(string=w972) -> (number=w948:dbl[])  [unwired: 3 in, 1 out]
        n272 = Concatenate Strings(w960, "-vsu2-" ("Substring"), w975, w939, ".txt" ("Substring")) -> (w973:string)
        n273 = String To Path(string=w973) -> (path=w964:path)
        n274 = Index Array(array=w948, index=1 ("Index")) -> (element=w947:dbl)
        n275 = Index Array(array=w948, index=0 ("Index")) -> (element=w945:dbl)
        n276 = call "4155C Config VSU2 Stress.vi"("error in (no error)"=w977, "VSU2"=w945, "Display on/off"=TRUE, "VISA session"=w978) -> ("error out"=w979:errorcluster, "dup VISA resource name"=w980:refnum<visa-resource-name>)
        n277 = call "4155C Apply Stress.vi"("error in (no error)"=w979, "Duration"=w947, "Emergency Stop"=w959, "VISA resource name in"=w980) -> ("error out"=w957:errorcluster, "VISA Resource Name out"=w955:refnum<visa-resource-name>)
        n278 = VISA Write(VISA resource name=w955, write buffer=":DISP ON" ("write buffer (\"\")"), error in (no error)=w957) -> (VISA resource name out=w954:refnum<visa-resource-name>, error out=w956:errorcluster)  [unwired: 1 out]
        n279 = call <vilib>:"compatOverwrite.vi"("overwrite (F)"=TRUE) -> ("overwrite?"=w944:T7)
        n280 = Open/Create/Replace File(file path (use dialog)=w964, error in=w956, operation (0:open)=w944) -> (refnum out=w967:refnum<file>, error out=w966:errorcluster)  [unwired: 3 in, 1 out]
        n281 = call "4155C Write array to file.vi"("Byte Stream File Refnum"=w967, "Header"=string[] ["VSU2 pulse completed successfully", ""], "error in (no error)"=w966) -> ("dup refnum"=w969:refnum<file>, "error out"=w968:errorcluster)  [unwired: 2 in]
        n282 = Close File(refnum=w969, error in=w968) -> (error out=w962:errorcluster)  [unwired: 1 out]
      }
      frame "sample-fpp" {
        w993 = string[] ["Time /s", "Id VgVd /A", "Ig VgVd /A", "Vp1 VgVd /V", "Vp2 VgVd /V"] ("Header")
        w997 = "%d" ("format string")
        n283 = Number To Decimal String(number=w982) -> (decimal integer string=w1045:string)  [unwired: 1 in]
        n284 = Fract/Exp String To Number(string=w1042) -> (number=w1030:dbl[])  [unwired: 3 in, 1 out]
        n285 = Concatenate Strings(w1036, "-samplefpp-" ("Substring"), w1045, w981, ".txt" ("Substring")) -> (w1043:string)
        n286 = String To Path(string=w1043) -> (path=w1005:path)
        n287 = Index Array(array=w1030, index=0 ("Index")) -> (element=w991:dbl)
        n288 = Index Array(array=w1030, index=1 ("Index")) -> (element=w990:dbl)
        n289 = Index Array(array=w1030, index=2 ("Index")) -> (element=w1038:dbl)
        n290 = Index Array(array=w1030, index=3 ("Index")) -> (element=w1028:dbl)
        n291 = call "4155C Config Sampling Measurements FPP.vi"("VISA session"=w1048, "Num Points"=w1038, "Vg"=w991, "Display on/off"=TRUE, "Gate Compliance"=w1037, "Drain Compliance"=w1046, "Standby"="Standby", "error in (no error)"=w1047, "Timings"=w1035, "Vd"=w990, "Sample time"=w1028) -> ("dup VISA resource name"=w1007:refnum<visa-resource-name>, "error out"=w1006:errorcluster)  [unwired: 3 in]
        n292 = Number To Decimal String(number=w991) -> (decimal integer string=w1017:string)  [unwired: 1 in]
        n293 = call "4155C Take Sample FPP.vi"("VISA resource name in"=w1007, "error in (no error)"=w1006, "Emergency Stop"=w1008) -> ("Time"=w1012:dbl[], "Vp1"=w1022:dbl[], "VISA Resource Name out"=w988:refnum<visa-resource-name>, "Ig"=w1010:dbl[], "Id"=w1011:dbl[], "Vp2"=w1020:dbl[], "error out"=w1009:errorcluster)  [unwired: 10 in]
        n294 = Insert Into Array(array=dbl[][] [] ("Input Array"), new element=w1012) -> (w1026:dbl[][])  [unwired: 2 in]
        n295 = Number To Decimal String(number=w990) -> (decimal integer string=w1015:string)  [unwired: 1 in]
        n296 = Insert Into Array(array=w1026, new element=w1011) -> (w1025:dbl[][])  [unwired: 2 in]
        n297 = Concatenate Strings("(Vg = " ("Substring"), w1017, "V, Vd = " ("Substring"), w1015, "V)" ("Substring")) -> (w1013:string)
        n298 = Insert Into Array(array=w1025, new element=w1010) -> (w1024:dbl[][])  [unwired: 2 in]
        n299 = Insert Into Array(array=w1024, new element=w1022) -> (w1021:dbl[][])  [unwired: 2 in]
        n300 = Insert Into Array(array=w1021, new element=w1020) -> (w989:dbl[][])  [unwired: 2 in]
        n301 = call <vilib>:"compatOverwrite.vi"("overwrite (F)"=TRUE) -> ("overwrite?"=w986:T7)
        n302 = Open/Create/Replace File(file path (use dialog)=w1005, error in=w1009, operation (0:open)=w986) -> (refnum out=w1002:refnum<file>, error out=w1003:errorcluster)  [unwired: 3 in, 1 out]
        n303 = Array To Spreadsheet String(array=w993, 3:w997) -> (spreadsheet string=w999:string)  [unwired: 1 in]
        n304 = Transpose 2D Array(2D array=w989) -> (transposed array=w1019:dbl[][])
        n305 = Search and Replace String(replace all?=TRUE ("replace all? (F)"), input string=w999, search string="VgVd", replace string=w1013) -> (result string=w995:string)  [unwired: 4 in, 3 out]
        n306 = Spreadsheet String To Array(format string=w997, spreadsheet string=w995, array type (2D Dbl)=w993) -> (array=w994:string[])  [unwired: 1 in]
        n307 = call "4155C Write array to file.vi"("Byte Stream File Refnum"=w1002, "Header"=w994, "Data Array"=w1019, "error in (no error)"=w1003) -> ("dup refnum"=w1000:refnum<file>, "error out"=w1001:errorcluster)  [unwired: 1 in]
        n308 = Close File(refnum=w1000, error in=w1001) -> (error out=w987:errorcluster)  [unwired: 1 out]
      }
      frame "resample-fpp" {
        w1063 = string[] ["Time /s", "Id VgVd /A", "Ig VgVd /A", "Vp1 VgVd /V", "Vp2 VgVd /V"] ("Header")
        w1067 = "%d" ("format string")
        n309 = Number To Decimal String(number=w1049) -> (decimal integer string=w1107:string)  [unwired: 1 in]
        n310 = Fract/Exp String To Number(string=w1104) -> (number=w1056:dbl[])  [unwired: 3 in, 1 out]
        n311 = Concatenate Strings(w1100, "-resamplefpp-" ("Substring"), w1107, w1050, ".txt" ("Substring")) -> (w1105:string)
        n312 = String To Path(string=w1105) -> (path=w1075:path)
        n313 = Index Array(array=w1056, index=0 ("Index")) -> (element=w1062:dbl)
        n314 = Index Array(array=w1056, index=1 ("Index")) -> (element=w1061:dbl)
        n315 = Number To Decimal String(number=w1062) -> (decimal integer string=w1085:string)  [unwired: 1 in]
        n316 = call "4155C Take Sample FPP.vi"("VISA resource name in"=w1058, "error in (no error)"=w1057, "Emergency Stop"=w1076) -> ("Time"=w1080:dbl[], "Vp1"=w1090:dbl[], "VISA Resource Name out"=w1060:refnum<visa-resource-name>, "Ig"=w1078:dbl[], "Id"=w1079:dbl[], "Vp2"=w1088:dbl[], "error out"=w1077:errorcluster)  [unwired: 10 in]
        n317 = Insert Into Array(array=dbl[][] [] ("Input Array"), new element=w1080) -> (w1094:dbl[][])  [unwired: 2 in]
        n318 = Number To Decimal String(number=w1061) -> (decimal integer string=w1083:string)  [unwired: 1 in]
        n319 = Insert Into Array(array=w1094, new element=w1079) -> (w1093:dbl[][])  [unwired: 2 in]
        n320 = Concatenate Strings("(Vg = " ("Substring"), w1085, "V, Vd = " ("Substring"), w1083, "V)" ("Substring")) -> (w1081:string)
        n321 = Insert Into Array(array=w1093, new element=w1078) -> (w1092:dbl[][])  [unwired: 2 in]
        n322 = Insert Into Array(array=w1092, new element=w1090) -> (w1089:dbl[][])  [unwired: 2 in]
        n323 = Insert Into Array(array=w1089, new element=w1088) -> (w1055:dbl[][])  [unwired: 2 in]
        n324 = call <vilib>:"compatOverwrite.vi"("overwrite (F)"=TRUE) -> ("overwrite?"=w1054:T7)
        n325 = Open/Create/Replace File(file path (use dialog)=w1075, error in=w1077, operation (0:open)=w1054) -> (refnum out=w1072:refnum<file>, error out=w1073:errorcluster)  [unwired: 3 in, 1 out]
        n326 = Array To Spreadsheet String(array=w1063, 3:w1067) -> (spreadsheet string=w1069:string)  [unwired: 1 in]
        n327 = Transpose 2D Array(2D array=w1055) -> (transposed array=w1087:dbl[][])
        n328 = Search and Replace String(replace all?=TRUE ("replace all? (F)"), input string=w1069, search string="VgVd", replace string=w1081) -> (result string=w1065:string)  [unwired: 4 in, 3 out]
        n329 = Spreadsheet String To Array(format string=w1067, spreadsheet string=w1065, array type (2D Dbl)=w1063) -> (array=w1064:string[])  [unwired: 1 in]
        n330 = call "4155C Write array to file.vi"("Byte Stream File Refnum"=w1072, "Header"=w1064, "Data Array"=w1087, "error in (no error)"=w1073) -> ("dup refnum"=w1070:refnum<file>, "error out"=w1071:errorcluster)  [unwired: 1 in]
        n331 = Close File(refnum=w1070, error in=w1071) -> (error out=w1059:errorcluster)  [unwired: 1 out]
      }
      frame "serial" {
        n332 = Index Array(array=w1111, index=0 ("Index")) -> (element=w1110:string)
        n333 = call "Serial write and read v0.4.vi"("Termination char\n(0xA = '\\n' = LF)\n(0xD = '\\r' = CR)"="Termination char\n(0xA = '\\n' = LF)\n(0xD = '\\r' = CR)", "Enable Termination\nChar (T)"="Enable Termination\nChar (T)", "parity"="parity", "stop bits"="stop bits", "string to write"=w1110, "flow control"="flow control", "byte count"="byte count", "Serial Settings:Serial End Mode for Reads"="Serial Settings:Serial End Mode for Reads", "Timeout (ms)"="Timeout (ms)", "error in (no error)"=w1116, "VISA resource name"="VISA resource name", "baud rate"="baud rate", "data bits"="data bits") -> ("read string"=→"Serial output":string, "error out"=w1115:errorcluster)  [unwired: 1 in]
      }
    }
  }
  "error out" <- w9
